vi "commander.vi"() -> ()   [LabVIEW 2012]
uses:
  <vilib>/Analysis/Matrix/Datatypes/RealMatrix.ctl
  G_VEH.vi
  G_SEN.vi
  G_PATH.vi
  G_DATA.vi
  G_LCM.vi
  <vilib>/Analysis/Matrix/Numeric/Conversions/Array To Matrix - RA2.vi
  <vilib>/Analysis/baseanly.llb/Real A x B.vi
  G_NAV.vi
  <vilib>/Analysis/Matrix/NI_Matrix.lvlib
  <vilib>/Analysis/NI_AALBase.lvlib
panel:
  in  "Boolean 2":bool
  out "Array":dbl[][](array[numeric])
  in  "Boolean":bool=TRUE
  out "LCM Recv Data":string
  out "GPS DATA 2":T1={"type"="None", "x_lcc"=-59.06772232055664, "y_lcc"=-26.082616806030273, "latdev"=0.0, "londev"=0.0, "sats"=0, "gps_l1_ranges"=0, "gps_l1_mask_ranges"=0, "gps_l2_mask_ranges"=0, "Heading"=89.78975677490234, "lon"=0.0, "lat"=0.0, "time"="None", "hgps"=89.78975677490234, "lag"=89.78975677490234, "MAP"="None"} {"lag" format="%#_5g"; "hgps" format="%#_5g"; "lat" format="%#_11g"; "lon" format="%#_11g"; "Heading" format="%#_5g"; "latdev" format="%#_4g"; "londev" format="%#_4g"}
  in  "LCM":bool
  in  "obs":bool
  in  "x":dbl
  in  "log":bool
  out "Waveform Chart 5":dbl(graph)
  in  "y":dbl min=-1.0 max=1.0 step=1.0
  out "x = 0?":bool
  out "timmer 2":u32
  out "timmer":u32
  out "Speed limit":dbl=8.0
  out "collision":bool
  out "Mission":i32=9
  in  "Load WPT":bool
  in  "Max. Vel.":dbl=20.0
  in  "RESET PATH":bool
  out "col":i16(graph)
  out "stop":bool
  in  "Reverse":bool
  in  "STOP":bool
  out "Waveform Chart 4":cluster{"auto":i16, "run":i16}(graph)={"auto"=1, "run"=0}
  out "Waveform Chart 3":T2(graph)={"Steer_input"=10.50986504720403, "Steer_output"=3.6, "handle"=10.50986504720403}
  out "Waveform Chart 2":T3(graph)={"VS_des"=4.606086314285715, "VS_can"=8.738, "VS_des"=5.0237113142857135}
  out "Heading":cluster{"Heading":dbl, "hgps":dbl}(graph)={"Heading"=269.76568785604456, "hgps"=270.2149981902155}
  out "XY Graph 2":cluster{"Y":dbl[], "Y":dbl[]}[](graph)=[{"Y"=[-241.57278442382812], "Y"=[-497.6172790527344]}, {"Y"=array[297 elements], "Y"=array[297 elements]}, {"Y"=array[297 elements], "Y"=array[297 elements]}, {"Y"=[-96.81030887093378], "Y"=[-438.1146154201037]}]
  out "Gauge":cluster{dbl, dbl, dbl}(knob)={4.606086314285715, 8.738, 5.0237113142857135} scale=-20.0..140.0
  out "Meter":cluster{dbl, dbl, dbl}(knob)={10.50986504720403, 3.6, 10.50986504720403} scale=-550.0..550.0
  out "XY Graph":cluster{"Y":dbl[], "Y":dbl[]}[](graph)=[{"Y"=[0.0], "Y"=[1000.0]}, {"Y"=[], "Y"=[]}, {"Y"=[], "Y"=[]}, {"Y"=[55.79381017995934], "Y"=[-143.41137512848826]}, {"Y"=[1.8243630881955273], "Y"=[-0.6091599202647308]}, {"Y"=[60.825233010671326, 56.37330625127248, 55.349089235151354, 59.801015994550255, 60.825233010671326], "Y"=[-144.72018116547483, -142.44414335187238, -144.44751039360185, -146.72354820720435, -144.72018116547483]}, {"Y"=[0.0, 2.210107140854234e-06, 8.840428449730098e-06, 1.9890964154001267e-05, 3.536171391260723e-05, 5.5252677611861145e-05, 7.956385525176302e-05, 0.00010829524660493917, 0.00014144685155770276, 0.0001790186695416196, 0.00022101070067037654, 0.00026742294460291305, 0.00031825540077079495, 0.00037350806894664856, 0.0004331809489031002, 0.0004972740399580289, 0.0005657873416566872, 0.0006387208537717015, 0.0007160745756209508, 0.0007978485066360008, 0.0008840426462484174, 0.0009746569938897665, 0.0010696915488779268, 0.0011691463105307776, 0.0012730212781661976, 0.001381316451102066, 0.0014940318285425747, 0.0016111674095782291, 0.0017327231935269083, 0.0018586991794791174, 0.001989095366525362, 0.00212391175364246, 0.002263148340148291, 0.0024068051247922995, 0.002554882106551304, 0.0027073792846294964, 0.002864296657776322, 0.003025634224741225, 0.003191391984614711, 0.0033615699362599116, 0.003536168078198898, 0.0037151864094084885, 0.003898624928524441, 0.004086483634296201, 0.004278762525359525, 0.004475461600350172, 0.0046765808579039, 0.004882120296656467, 0.0050920799150162566, 0.00530645971150534, 0.005525259684645789, 0.005748479832959674, 0.005976120154741693, 0.006208180648513917, 0.006444661312457356, 0.006685562145094082, 0.006930883144491418, 0.007180624309171435, 0.007434785636974084, 0.007693367126535122, 0.007956368775921874, 0.008223790583087975, 0.008495632546100751, 0.008771894663368585, 0.009052576932504053, 0.00933767935191554, 0.009627201919329309, 0.009921144632812684, 0.010219507490205615, 0.010522290489461739, 0.010829493628421005, 0.011141116904923365, 0.011457160316581394, 0.011777623861462416, 0.012102507536951634, 0.012431811341116372, 0.012765535271228146, 0.013103679325240591, 0.0134462435006526, 0.013793227794963059, 0.014144632205784546, 0.014500456730615952, 0.014860701366956164, 0.015225366112190386, 0.015594450963703821, 0.015967955919109045, 0.0163458809754502, 0.016728226130226176, 0.017114991380822175, 0.017506176724168654, 0.0179017821577645, 0.018301807678767545, 0.018706253284335617, 0.019115118971512857, 0.019528404737457095, 0.01994611057932616, 0.02036823649393682, 0.02079478247856059, 0.021225748530014243, 0.02166113464522823, 0.022100940821246695], "Y"=[0.0, 0.05249999993797367, 0.10499999950378934, 0.15749999832528905, 0.2099999960303148, 0.26249999224670867, 0.31499998660231265, 0.3674999787249688, 0.41999996824251923, 0.472499954782806, 0.5249999379736712, 0.577499917442957, 0.6299998928185055, 0.682499863728159, 0.7349998297997596, 0.7874997906611497, 0.8399997459401715, 0.8924996952646672, 0.9449996382624795, 0.9974995745614504, 1.0499995037894228, 1.1024994255742389, 1.1549993395437415, 1.2074992453257731, 1.2599991425481762, 1.3124990308387938, 1.3649989098254687, 1.4174987791360436, 1.4699986383983614, 1.5224984872402658, 1.574998325289599, 1.6274981521742047, 1.6799979675219257, 1.7324977709606055, 1.784997562118088, 1.837497340622216, 1.8899971061008334, 1.9424968581817836, 1.994996596492911, 2.047496320662059, 2.099996030317072, 2.152495725085793, 2.204995404596067, 2.2574950684757384, 2.309994716352652, 2.3624943478546507, 2.414993962609581, 2.467493560245286, 2.519993140389611, 2.5724927026704023, 2.6249922467155042, 2.6774917721527607, 2.7299912786100196, 2.7824907657151243, 2.834990233095921, 2.887489680380256, 2.939989107195975, 2.9924885131709242, 3.0449878979329497, 3.0974872611098974, 3.1499866023296144, 3.2024859212199472, 3.2549852174087435, 3.3074844905238483, 3.3599837401931105, 3.412482966044377, 3.464982167705495, 3.5174813448043127, 3.5699804969686775, 3.6224796238264374, 3.6749787250054404, 3.7274778001335362, 3.7799768488385714, 3.8324758707483966, 3.884974865490859, 3.9374738326938097, 3.989972771985096, 4.042471682992569, 4.094970565344078, 4.147469418667473, 4.199968242590603, 4.2524670367413195, 4.304965800747474, 4.3574645342369145, 4.409963236837495, 4.4624619081770645, 4.514960547883476, 4.567459155584579, 4.6199577309082285, 4.672456273482274, 4.724954782934569, 4.777453258892966, 4.829951700985317, 4.882450108839476, 4.934948482083297, 4.987446820344632, 5.039945123251335, 5.09244339043126, 5.144941621512262, 5.197439816122197, 5.249937973888915]}, {"Y"=[55.85492946607054, 56.300112183962334, 56.74529490185413, 57.19047761974598, 57.635660337637766, 58.08084305552956, 58.52602577342136, 58.97120849131315, 59.416391209205, 59.8615739270968, 60.306756644988596, 60.75193936288038, 61.197122080772175, 61.64230479866403, 62.087487516555825, 62.532670234447615, 62.97785295233941, 63.423035670231265, 63.86821838812306, 64.31340110601485, 64.75858382390665, 65.20376654179844, 65.64894925969023, 66.09413197758208, 66.53931469547388, 66.98449741336567, 67.42968013125746, 67.87486284914931, 68.3200455670411, 68.7652282849329, 69.2104110028247, 69.65559372071655, 70.10077643860835, 70.54595915650015, 70.99114187439193, 71.43632459228371, 71.88150731017556, 72.32669002806736, 72.77187274595916, 73.21705546385095], "Y"=[-143.26925304077835, -143.49687629901547, -143.72449955725253, -143.95212281548962, -144.17974607372668, -144.40736933196374, -144.63499259020085, -144.8626158484379, -145.090239106675, -145.3178623649121, -145.54548562314918, -145.7731088813862, -146.00073213962332, -146.22835539786038, -146.45597865609744, -146.68360191433456, -146.91122517257162, -147.1388484308087, -147.36647168904577, -147.59409494728285, -147.82171820551994, -148.04934146375703, -148.27696472199406, -148.50458798023115, -148.73221123846827, -148.9598344967053, -149.18745775494241, -149.4150810131795, -149.64270427141656, -149.87032752965362, -150.09795078789074, -150.3255740461278, -150.55319730436486, -150.78082056260195, -151.00844382083903, -151.23606707907612, -151.46369033731318, -151.6913135955503, -151.91893685378736, -152.14656011202442]}, {"Y"=[46.95734422441421, 47.0463827596022, 47.13542129479015, 47.224459829978144, 47.31349836516614, 47.40253690035408, 47.49157543554208, 47.58061397073008, 47.669652505918016, 47.75869104110601, 47.84772957629395, 47.936768111481946, 48.02580664666995, 48.11484518185789, 48.20388371704588, 48.292922252233886, 48.381960787421825, 48.47099932260982, 48.56003785779782, 48.64907639298576, 48.73811492817376, 48.827153463361746, 48.91619199854969, 49.00523053373769, 49.09426906892568, 49.18330760411363, 49.272346139301625, 49.361384674489564, 49.45042320967757, 49.53946174486556, 49.6285002800535, 49.717538815241504, 49.8065773504295, 49.89561588561743, 49.984654420805434, 50.07369295599343, 50.16273149118137, 50.251770026369364, 50.34080856155737, 50.429847096745306, 50.5188856319333, 50.607924167121304, 50.69696270230924, 50.78600123749724, 50.875039772685184, 50.96407830787318, 51.05311684306117, 51.142155378249115, 51.23119391343711, 51.320232448625106, 51.40927098381305, 51.49830951900105, 51.58734805418904, 51.67638658937698, 51.765425124564985, 51.85446365975298, 51.94350219494092, 52.03254073012892, 52.12157926531691, 52.21061780050485, 52.29965633569285, 52.38869487088079, 52.477733406068786, 52.56677194125679, 52.65581047644473, 52.74484901163272, 52.833887546820726, 52.922926082008665, 53.01196461719666, 53.10100315238466, 53.190041687572595, 53.27908022276059, 53.36811875794859, 53.45715729313653, 53.54619582832453, 53.635234363512524, 53.72427289870047, 53.813311433888465, 53.902349969076404, 53.99138850426441, 54.0804270394524, 54.16946557464034, 54.25850410982834, 54.34754264501633, 54.43658118020427, 54.525619715392274, 54.61465825058027, 54.70369678576821, 54.792735320956204, 54.88177385614421, 54.970812391332146, 55.05985092652014, 55.148889461708144, 55.23792799689608, 55.32696653208408, 55.41600506727202, 55.50504360246001, 55.59408213764801, 55.683120672835955, 55.77215920802395, 55.861197743211946, 55.95023627839994, 56.03927481358789, 56.12831334877588, 56.21735188396388, 56.306390419151825, 56.39542895433982, 56.48446748952781, 56.573506024715755, 56.66254455990375, 56.75158309509169, 56.84062163027969, 56.92966016546769, 57.01869870065563, 57.10773723584363, 57.196775771031625, 57.285814306219564, 57.37485284140757, 57.46389137659556, 57.552929911783494, 57.64196844697149, 57.73100698215949, 57.82004551734743, 57.90908405253543, 58.08716112291137, 58.176199658099364, 58.26523819328731, 58.354276728475305, 58.4433152636633, 58.53235379885125, 58.62139233403924, 58.71043086922723, 58.79946940441518, 58.88850793960317, 58.97754647479111, 59.06658500997911, 59.15562354516711, 59.24466208035505, 59.333700615543044, 59.42273915073105, 59.511777685918986, 59.60081622110698, 59.689854756294984, 59.778893291482916, 59.86793182667091, 59.956970361858914, 60.04600889704685, 60.13504743223485, 60.31312450261079, 60.402163037798786, 60.491201572986725, 60.58024010817473, 60.66927864336272, 60.75831717855066, 60.84735571373866, 60.93639424892665, 61.02543278411459, 61.114471319302595, 61.203509854490534, 61.29254838967853, 61.38158692486653, 61.47062546005447, 61.55966399524247, 61.64870253043047, 61.73774106561841, 61.826779600806404, 61.91581813599439, 62.00485667118234, 62.093895206370334, 62.18293374155833, 62.271972276746276, 62.36101081193427, 62.45004934712227, 62.53908788231021, 62.62812641749821, 62.71716495268615, 62.80620348787415, 62.895242023062146, 62.984280558250084, 63.07331909343808, 63.162357628626076, 63.251396163814015, 63.34043469900201, 63.42947323419001, 63.51851176937796, 63.60755030456595, 63.69658883975394, 63.78562737494189, 63.87466591012988, 63.96370444531783, 64.05274298050581, 64.14178151569382, 64.23082005088176, 64.31985858606976, 64.40889712125775, 64.4979356564457, 64.58697419163369, 64.76505126200964, 64.85408979719762, 64.94312833238557, 65.03216686757357, 65.12120540276156, 65.2102439379495, 65.29928247313751, 65.38832100832549, 65.47735954351344, 65.56639807870144, 65.65543661388938, 65.74447514907737, 65.83351368426537, 65.92255221945331, 66.0115907546413, 66.10062928982931, 66.18966782501724, 66.27870636020525, 66.36774489539324, 66.45678343058118, 66.54582196576918, 66.63486050095719, 66.72389903614511, 66.81293757133312, 66.9019761065211, 66.99101464170904, 67.08005317689705, 67.16909171208498, 67.25813024727299, 67.34716878246098, 67.43620731764892, 67.52524585283692, 67.61428438802493, 67.70332292321285, 67.79236145840086, 67.88139999358886, 67.97043852877678, 68.05947706396479, 68.14851559915279, 68.23755413434073, 68.32659266952872, 68.41563120471668, 68.50466973990466, 68.59370827509267, 68.6827468102806, 68.7717853454686, 68.8608238806566, 68.94986241584455, 69.03890095103253, 69.12793948622053, 69.21697802140848, 69.30601655659646, 69.39505509178447, 69.48409362697241, 69.5731321621604, 69.6621706973484, 69.75120923253635, 69.84024776772434, 69.92928630291229, 70.01832483810027, 70.10736337328828, 70.19640190847622, 70.2854404436642, 70.37447897885221, 70.46351751404015, 70.55255604922814, 70.64159458441614, 70.7306331196041, 70.81967165479207, 70.90871018998008, 70.99774872516802, 71.08678726035602, 71.17582579554401, 71.26486433073195, 71.35390286591995, 71.44294140110789, 71.5319799362959, 71.62101847148388, 71.71005700667183, 71.79909554185983, 71.88813407704782, 71.97717261223576, 72.06621114742377, 72.15524968261175, 72.2442882177997, 72.3333267529877, 72.42236528817568, 72.51140382336364, 72.60044235855163, 72.68948089373963, 72.77851942892757, 72.86755796411556, 72.9565964993035, 73.04563503449151, 73.13467356967949, 73.22371210486745, 73.31275064005544, 73.40178917524342, 73.49082771043138, 73.57986624561937], "Y"=[-138.89375124553214, -138.93927200180423, -138.98479275807625, -139.0303135143483, -139.07583427062036, -139.12135502689242, -139.16687578316444, -139.21239653943653, -139.25791729570855, -139.30343805198058, -139.34895880825266, -139.3944795645247, -139.44000032079677, -139.4855210770688, -139.53104183334085, -139.5765625896129, -139.62208334588496, -139.667604102157, -139.71312485842907, -139.7586456147011, -139.80416637097318, -139.8496871272452, -139.89520788351723, -139.9407286397893, -139.98624939606134, -140.0317701523334, -140.07729090860545, -140.1228116648775, -140.16833242114956, -140.2138531774216, -140.25937393369364, -140.30489468996572, -140.35041544623775, -140.39593620250977, -140.44145695878186, -140.48697771505388, -140.53249847132597, -140.578019227598, -140.62353998387005, -140.66906074014207, -140.71458149641416, -140.76010225268618, -140.80562300895826, -140.8511437652303, -140.89666452150234, -140.9421852777744, -140.98770603404643, -141.0332267903185, -141.07874754659053, -141.1242683028626, -141.16978905913462, -141.2153098154067, -141.26083057167872, -141.3063513279508, -141.35187208422283, -141.3973928404949, -141.44291359676694, -141.48843435303897, -141.53395510931105, -141.57947586558308, -141.62499662185516, -141.67051737812716, -141.71603813439924, -141.76155889067127, -141.80707964694335, -141.85260040321535, -141.89812115948743, -141.94364191575949, -141.9891626720315, -142.0346834283036, -142.08020418457562, -142.1257249408477, -142.1712456971197, -142.21676645339178, -142.2622872096638, -142.3078079659359, -142.3533287222079, -142.39884947847997, -142.44437023475203, -142.48989099102408, -142.53541174729614, -142.58093250356816, -142.62645325984025, -142.67197401611224, -142.71749477238433, -142.76301552865635, -142.80853628492844, -142.85405704120046, -142.89957779747255, -142.94509855374454, -142.99061931001663, -143.03614006628868, -143.0816608225607, -143.1271815788328, -143.17270233510482, -143.2182230913769, -143.2637438476489, -143.30926460392098, -143.354785360193, -143.4003061164651, -143.4458268727371, -143.4913476290092, -143.5368683852812, -143.58238914155328, -143.62790989782533, -143.67343065409736, -143.71895141036944, -143.76447216664147, -143.80999292291352, -143.85551367918555, -143.90103443545763, -143.94655519172966, -143.99207594800174, -144.03759670427374, -144.08311746054582, -144.12863821681785, -144.1741589730899, -144.21967972936199, -144.265200485634, -144.3107212419061, -144.3562419981781, -144.40176275445017, -144.4472835107222, -144.49280426699428, -144.58384577953836, -144.6293665358104, -144.67488729208247, -144.72040804835453, -144.76592880462653, -144.81144956089864, -144.85697031717064, -144.90249107344272, -144.94801182971474, -144.99353258598683, -145.03905334225882, -145.0845740985309, -145.13009485480293, -145.17561561107502, -145.22113636734704, -145.2666571236191, -145.31217787989118, -145.35769863616318, -145.40321939243526, -145.4487401487073, -145.49426090497937, -145.5397816612514, -145.58530241752348, -145.63082317379548, -145.7218646863396, -145.76738544261164, -145.8129061988837, -145.85842695515572, -145.90394771142783, -145.94946846769983, -145.9949892239719, -146.04050998024394, -146.08603073651602, -146.13155149278802, -146.1770722490601, -146.22259300533213, -146.2681137616042, -146.31363451787624, -146.3591552741483, -146.40467603042035, -146.45019678669237, -146.49571754296446, -146.54123829923648, -146.58675905550857, -146.6322798117806, -146.67780056805265, -146.72332132432467, -146.76884208059676, -146.81436283686878, -146.85988359314084, -146.9054043494129, -146.95092510568492, -146.99644586195703, -147.04196661822903, -147.0874873745011, -147.13300813077313, -147.17852888704522, -147.22404964331722, -147.2695703995893, -147.31509115586132, -147.3606119121334, -147.40613266840543, -147.4516534246775, -147.49717418094954, -147.54269493722157, -147.58821569349365, -147.63373644976568, -147.67925720603776, -147.72477796230976, -147.77029871858184, -147.81581947485387, -147.86134023112595, -147.90686098739798, -147.9979024999421, -148.0434232562141, -148.08894401248617, -148.13446476875822, -148.17998552503028, -148.22550628130233, -148.27102703757438, -148.3165477938464, -148.3620685501185, -148.40758930639052, -148.45311006266255, -148.49863081893463, -148.54415157520666, -148.58967233147874, -148.63519308775076, -148.6807138440228, -148.72623460029487, -148.77175535656693, -148.81727611283895, -148.86279686911104, -148.90831762538306, -148.95383838165512, -148.99935913792717, -149.0448798941992, -149.09040065047128, -149.1359214067433, -149.18144216301536, -149.22696291928742, -149.27248367555944, -149.31800443183153, -149.36352518810358, -149.4090459443756, -149.4545667006477, -149.50008745691972, -149.54560821319174, -149.59112896946382, -149.63664972573585, -149.68217048200793, -149.72769123827996, -149.77321199455199, -149.81873275082407, -149.86425350709612, -149.90977426336815, -149.95529501964023, -150.00081577591226, -150.0463365321843, -150.09185728845637, -150.1373780447284, -150.18289880100048, -150.2284195572725, -150.27394031354456, -150.3194610698166, -150.36498182608864, -150.4105025823607, -150.45602333863278, -150.5015440949048, -150.54706485117688, -150.5925856074489, -150.63810636372094, -150.68362711999302, -150.72914787626505, -150.7746686325371, -150.82018938880915, -150.86571014508118, -150.91123090135326, -150.9567516576253, -151.00227241389734, -151.04779317016943, -151.09331392644145, -151.13883468271348, -151.18435543898556, -151.2298761952576, -151.27539695152967, -151.3209177078017, -151.36643846407375, -151.4119592203458, -151.45747997661783, -151.5030007328899, -151.54852148916194, -151.594042245434, -151.63956300170608, -151.6850837579781, -151.73060451425013, -151.77612527052221, -151.82164602679424, -151.8671667830663, -151.91268753933835, -151.95820829561038, -152.00372905188246, -152.04924980815449, -152.09477056442654, -152.14029132069862, -152.18581207697065, -152.23133283324267, -152.27685358951476, -152.32237434578678, -152.36789510205887, -152.4134158583309, -152.45893661460295, -152.504457370875]}, {"Y"=[], "Y"=[]}, {"Y"=[], "Y"=[]}, {"Y"=[], "Y"=[]}, {"Y"=[-16.5, -15.25, -15.0, -13.5, -13.25, -13.25, -13.25, -13.0, -13.0, -12.75, -12.75, -12.75, -12.75, -12.75, -12.75, -12.75, -12.5, -12.5, -12.5, -12.5, -12.5, -12.5, -12.25, -12.25, -12.25, -12.25, -12.25, -12.25, -12.0, -12.0, -12.0, -11.75, -11.75, -11.75, -11.5, -11.5, -11.5, -11.5, -11.5, -11.25, -10.75, -10.75, -10.5, -10.5, -10.25, -10.25, -10.0, -10.0, -10.0, -10.0, -10.0, -9.75, -9.75, -9.75, -9.75, -9.75, -9.75, -9.75, -9.75, -9.75, -9.75, -9.5, -9.5, -9.5, -9.5, -9.5, -9.5, -9.5, -9.5, -9.5, -9.5, -9.5, -9.5, -9.5, -9.5, -9.5, -9.5, -9.5, -9.5, -9.5, -9.25, -9.25, -9.25, -9.25, -9.25, -9.25, -9.25, -9.25, -9.25, -9.25, -9.25, -9.25, -9.25, -9.25, -9.25, -9.25, -9.25, -9.25, -9.25, -9.25, -9.25, -9.25, -9.0, -9.0, -9.0, -9.0, -9.0, -9.0, -9.0, -9.0, -9.0, -9.0, -9.0, -9.0, -9.0, -9.0, -9.0, -9.0, -9.0, -9.0, -9.0, -9.0, -9.0, -9.0, -9.0, -9.0, -9.0, -9.0, -8.75, -8.75, -8.75, -8.75, -8.75, -8.75, -8.75, -8.75, -8.75, -8.75, -8.75, -8.75, -8.75, -8.75, -8.75, -8.75, -8.75, -8.75, -8.75, -8.75, -8.75, -8.75, -8.75, -8.75, -8.75, -8.75, -8.75, -8.75, -8.75, -8.75, -8.75, -8.75, -8.75, -8.75, -8.75, -8.75, -8.75, -8.5, -8.5, -8.5, -8.5, -8.5, -8.5, -8.5, -8.5, -8.5, -8.5, -8.5, -8.5, -8.5, -8.5, -8.5, -8.5, -8.5, -8.5, -8.5, -8.5, -8.5, -8.5, -8.5, -8.5, -8.5, -8.5, -8.5, -8.5, -8.5, -8.5, -8.5, -8.5, -8.5, -8.5, -8.5, -8.5, -8.25, -8.25, -8.25, -8.25, -8.25, -8.25, -8.25, -8.25, -8.25, -8.25, -8.25, -8.25, -8.25, -8.25, -8.25, -8.25, -8.25, -8.25, -8.25, -8.25, -8.25, -8.25, -8.25, -8.25, -8.25, -8.25, -8.25, -8.25, -8.25, -8.25, -8.25, -8.25, -8.25, -8.0, -8.0, -8.0, -8.0, -8.0, -8.0, -8.0, -8.0, -8.0, -8.0, -8.0, -8.0, -8.0, -8.0, -8.0, -8.0, -8.0, -8.0, -8.0, -8.0, -8.0, -8.0, -8.0, -8.0, -8.0, -7.75, -7.75, -7.75, -7.75, -7.75, -7.75, -7.75, -7.75, -7.75, -7.75, -7.75, -7.75, -7.75, -7.75, -7.75, -7.75, -7.75, -7.75, -7.75, -7.75, -7.75, -7.75, -7.75, -7.75, -7.75, -7.75, -7.5, -7.5, -7.5, -7.5, -7.5, -7.5, -7.5, -7.5, -7.5, -7.5, -7.5, -7.5, -7.5, -7.5, -7.5, -7.5, -7.5, -7.5, -7.5, -7.5, -7.5, -7.5, -7.5, -7.5, -7.5, -7.25, -7.25, -7.25, -7.25, -7.25, -7.25, -7.25, -7.25, -7.25, -7.25, -7.25, -7.25, -7.25, -7.25, -7.25, -7.25, -7.25, -7.25, -7.25, -7.25, -7.25, -7.25, -7.25, -7.0, -7.0, -7.0, -7.0, -7.0, -7.0, -7.0, -7.0, -7.0, -7.0, -7.0, -7.0, -7.0, -7.0, -7.0, -7.0, -7.0, -7.0, -7.0, -6.75, -6.75, -6.75, -6.75, -6.75, -6.75, -6.75, -6.75, -6.75, -6.75, -6.75, -6.75, -6.75, -6.75, -6.75, -6.75, -6.75, -6.75, -6.75, -6.75, -6.75, -6.75, -6.75, -6.5, -6.5, -6.5, -6.5, -6.5, -6.5, -6.5, -6.5, -6.5, -6.5, -6.5, -6.5, -6.5, -6.5, -6.5, -6.5, -6.5, -6.5, -6.5, -6.5, -6.5, -6.5, -6.5, -6.5, -6.5, -6.5, -6.5, -6.5, -6.5, -6.5, -6.25, -6.25, -6.25, -6.25, -6.25, -6.25, -6.25, -6.25, -6.25, -6.25, -6.25, -6.25, -6.25, -6.25, -6.25, -6.25, -6.25, -6.0, -6.0, -6.0, -6.0, -6.0, -6.0, -6.0, -6.0, -6.0, -6.0, -6.0, -5.75, -5.75, -5.75, -5.75, -5.75, -5.75, -5.75, -5.75, -5.75, -5.75, -5.5, -5.25, -5.0, -4.75, -4.5, -4.5, -4.25, -4.25, -4.0, -4.0, -3.75, -3.75, -3.5, -3.5, -3.25, -3.25, -3.25, -3.25, -3.0, -3.0, 2.0, 2.0, 2.0, 2.0, 2.0, 2.0, 2.0, 2.25, 2.25, 2.25, 2.25, 2.25, 2.25, 2.25, 2.25, 2.25, 2.25, 2.25, 2.25, 2.25, 2.25, 2.25, 2.25, 2.25, 2.25, 2.25, 2.25, 2.25, 2.25, 2.5, 2.5, 2.5, 2.5, 2.5, 2.5, 2.5, 2.5, 2.5, 2.5, 2.5, 2.5, 2.5, 2.5, 2.5, 2.5, 2.5, 2.5, 2.5, 2.5, 2.5, 2.5, 2.5, 2.5, 2.5, 2.5, 2.5, 2.5, 2.5, 2.5, 2.5, 2.5, 2.5, 2.5, 2.5, 2.5, 2.5, 2.5, 2.5, 2.5, 2.5, 2.5, 2.75, 2.75, 2.75, 2.75, 2.75, 2.75, 2.75, 2.75, 2.75, 2.75, 2.75, 2.75, 2.75, 2.75, 2.75, 2.75, 2.75, 2.75, 2.75, 2.75, 2.75, 2.75, 2.75, 2.75, 2.75, 2.75, 2.75, 2.75, 2.75, 2.75, 2.75, 2.75, 2.75, 2.75, 2.75, 2.75, 2.75, 2.75, 2.75, 2.75, 2.75, 2.75, 2.75, 2.75, 2.75, 2.75, 2.75, 2.75, 2.75, 2.75, 3.0, 3.0, 3.0, 3.0, 3.0, 3.0, 3.0, 3.0, 3.0, 3.0, 3.0, 3.0, 3.0, 3.0, 3.0, 3.0, 3.0, 3.0, 3.0, 3.0, 3.0, 3.0, 3.0, 3.0, 3.0, 3.0, 3.0, 3.0, 3.0, 3.0, 3.0, 3.0, 3.0, 3.0, 3.0, 3.0, 3.0, 3.0, 3.0, 3.0, 3.0, 3.0, 3.0, 3.0, 3.0, 3.0, 3.0, 3.25, 3.25, 3.25, 3.25, 3.25, 3.25, 3.25, 3.25, 3.25, 3.25, 3.25, 3.25, 3.25, 3.25, 3.25, 3.25, 3.25, 3.25, 3.25, 3.25, 3.25, 3.25, 3.25, 3.25, 3.25, 3.25, 3.25, 3.25, 3.25, 3.25, 3.25, 3.25, 3.25, 3.25, 3.25, 3.25, 3.25, 3.25, 3.25, 3.25, 3.25, 3.25, 3.25, 3.25, 3.25, 3.25, 3.25, 3.25, 3.25, 3.25, 3.25, 3.25, 3.25, 3.5, 3.5, 3.5, 3.5, 3.5, 3.5, 3.5, 3.5, 3.5, 3.5, 3.5, 3.5, 3.5, 3.5, 3.5, 3.5, 3.5, 3.5, 3.5, 3.5, 3.5, 3.5, 3.5, 3.5, 3.5, 3.5, 3.5, 3.5, 3.5, 3.5, 3.5, 3.5, 3.5, 3.5, 3.5, 3.5, 3.5, 3.5, 3.5, 3.5, 3.5, 3.5, 3.5, 3.5, 3.5, 3.5, 3.5, 3.5, 3.5, 3.5, 3.5, 3.5, 3.5, 3.5, 3.5, 3.5, 3.5, 3.75, 3.75, 3.75, 3.75, 3.75, 3.75, 3.75, 3.75, 3.75, 3.75, 3.75, 3.75, 3.75, 3.75, 3.75, 3.75, 3.75, 3.75, 3.75, 3.75, 3.75, 3.75, 3.75, 3.75, 3.75, 3.75, 3.75, 3.75, 3.75, 3.75, 3.75, 3.75, 3.75, 3.75, 3.75, 3.75, 3.75, 4.0, 4.0, 4.0, 4.0, 4.0, 4.0, 4.0, 4.0, 4.0, 4.0, 4.0, 4.0, 4.0, 4.0, 4.0, 4.0, 4.0, 4.0, 4.0, 4.0, 4.0, 4.0, 4.0, 4.0, 4.0, 4.0, 4.0, 4.0, 4.0, 4.0, 4.0, 4.0, 4.0, 4.0, 4.0, 4.0, 4.25, 4.25, 4.25, 4.25, 4.25, 4.25, 4.25, 4.25, 4.25, 4.25, 4.25, 4.25, 4.25, 4.25, 4.25, 4.25, 4.25, 4.25, 4.25, 4.25, 4.25, 4.25, 4.25, 4.25, 4.25, 4.25, 4.25, 4.25, 4.25, 4.25, 4.25, 4.25, 4.25, 4.25, 4.25, 4.25, 4.25, 4.25, 4.25, 4.25, 4.25, 4.25, 4.25, 4.5, 4.5, 4.5, 4.5, 4.5, 4.5, 4.5, 4.5, 4.5, 4.5, 4.5, 4.5, 4.5, 4.5, 4.5, 4.5, 4.5, 4.5, 4.5, 4.5, 4.5, 4.5, 4.5, 4.5, 4.5, 4.5, 4.5, 4.75, 4.75, 4.75, 4.75, 4.75, 4.75, 4.75, 4.75, 4.75, 4.75, 4.75, 4.75, 4.75, 4.75, 4.75, 4.75, 4.75, 4.75, 4.75, 4.75, 4.75, 4.75, 4.75, 4.75, 4.75, 4.75, 4.75, 4.75, 4.75, 5.0, 5.0, 5.0, 5.0, 5.0, 5.0, 5.0, 5.0, 5.0, 5.0, 5.0, 5.0, 5.0, 5.0, 5.0, 5.0, 5.0, 5.0, 5.0, 5.0, 5.0, 5.25, 5.25, 5.25, 5.25, 5.25, 5.25, 5.25, 5.25, 5.25, 5.25, 5.25, 5.25, 5.25, 5.25, 5.5, 5.5, 5.5, 5.5, 5.5, 5.5, 5.5, 5.5, 5.5, 5.5, 5.5, 5.5, 5.75, 5.75, 5.75, 5.75, 5.75, 5.75, 5.75, 5.75, 5.75, 5.75, 5.75, 5.75, 5.75, 5.75, 5.75, 5.75, 5.75, 6.0, 6.0, 6.0, 6.0, 6.0, 6.0, 6.0, 6.0, 6.0, 6.0, 6.0, 6.25, 6.25, 6.25, 6.25, 6.25, 6.25, 6.25, 6.25, 6.5, 6.5, 6.5, 6.5, 6.5, 6.5, 6.5, 6.5, 6.5, 6.75, 6.75, 6.75, 6.75, 7.0, 7.0, 7.0, 7.25, 7.25, 7.25, 7.25, 7.25, 7.25, 7.25, 7.5, 7.5, 8.0, 8.0, 8.0, 8.0, 8.0, 8.25, 8.25, 8.5, 8.5, 8.5, 8.75, 8.75, 8.75, 8.75, 8.75, 9.0, 9.0, 9.0, 9.0, 9.0, 9.0, 9.25, 9.25, 9.25, 9.25, 9.25, 9.25, 9.5, 9.5, 9.5, 9.5, 9.5, 9.5, 9.75, 9.75, 9.75, 10.0, 10.0, 10.0, 10.0, 10.25, 10.25, 10.5, 10.5, 10.5, 10.75, 10.75, 10.75, 10.75, 11.0, 11.0, 11.0, 11.0, 11.0, 11.25, 11.25, 11.25, 11.25, 11.25, 11.25, 11.25, 11.25, 11.25, 11.25, 11.5, 11.5, 11.5, 11.5, 11.5, 11.5, 11.5, 11.5, 11.5, 11.5, 11.5, 11.5, 11.5, 11.5, 11.5, 11.75, 11.75, 11.75, 11.75, 11.75, 11.75, 11.75, 11.75, 11.75, 11.75, 11.75, 11.75, 11.75, 11.75, 11.75, 11.75, 11.75, 11.75, 11.75, 11.75, 12.0, 12.0, 12.0, 12.0, 12.0, 12.0, 12.0, 12.0, 12.0, 12.0, 12.0, 12.0, 12.0, 12.0, 12.0, 12.0, 12.0, 12.0, 12.0, 12.0, 12.0, 12.0, 12.0, 12.0, 12.0, 12.0, 12.0, 12.25, 12.25, 12.25, 12.25, 12.25, 12.25, 12.25, 12.25, 12.25, 12.25, 12.25, 12.25, 12.25, 12.25, 12.25, 12.25, 12.5, 12.5, 12.5, 12.5, 12.5, 12.5, 12.5, 12.5, 12.5, 12.5, 12.5, 12.5, 12.5, 12.75, 12.75, 12.75, 12.75, 12.75, 12.75, 12.75, 12.75, 12.75, 12.75, 13.0, 13.0, 13.0, 13.0, 13.0, 13.0, 13.0, 13.0, 13.0, 13.0, 13.0, 13.0, 13.0, 13.0, 13.0, 13.0, 13.0, 13.0, 13.0, 13.0, 13.0, 13.0, 13.0, 13.25, 13.25, 13.25, 13.25, 13.25, 13.25, 13.25, 13.25, 13.25, 13.25, 13.25, 13.25, 13.25, 13.25, 13.25, 13.25, 13.25, 13.25, 13.25, 13.5, 13.5, 13.5, 13.5, 13.5, 13.5, 13.5, 13.5, 13.5, 13.5, 13.75, 13.75, 13.75, 13.75, 13.75, 13.75, 13.75, 13.75, 13.75, 14.0, 14.0, 14.0, 14.0, 14.5, 14.75, 15.5, 15.75, 16.0, 19.25, 19.25, 19.25, 19.5, 19.5, 19.75, 22.25, 22.25, 22.25, 22.5, 22.5, 22.5, 22.75, 22.75, 22.75, 22.75, 23.0, 23.0, 23.0, 23.25, 23.25, 23.25, 23.5, 23.5, 23.5, 23.5, 23.5, 23.5, 23.75, 23.75, 23.75, 23.75, 23.75, 23.75, 23.75, 23.75, 23.75, 23.75, 23.75, 24.0, 24.0, 24.0, 24.0, 24.0, 24.0, 24.0, 24.25, 24.25, 24.5], "Y"=[46.5, 46.5, 46.5, 2.75, 0.5, 2.75, 17.0, 0.75, 17.25, -6.5, -2.25, -1.75, 0.5, 0.75, 1.0, 3.75, -6.5, 0.75, 4.0, 4.25, 17.25, 21.5, -6.75, -6.5, -1.75, 17.25, 21.5, 22.25, -6.75, 21.75, 22.0, -6.5, 11.25, 22.0, 10.5, 10.75, 11.0, 11.5, 11.75, -6.0, 3.75, 8.25, -1.0, 8.25, -1.25, -1.0, -7.0, -1.25, 2.75, 3.0, 3.5, -10.75, -10.5, -10.0, -9.5, -9.25, -8.25, -6.75, -1.25, 3.0, 3.25, -20.5, -15.5, -15.25, -14.75, -10.5, -10.25, -10.0, -9.75, -9.25, -9.0, -8.75, -8.25, -8.0, -7.75, -7.5, -1.0, 0.5, 1.5, 2.75, -20.25, -18.25, -17.75, -17.5, -17.0, -15.75, -15.5, -10.75, -10.25, -9.5, -9.0, -8.75, -8.25, -8.0, -7.75, 0.75, 1.0, 1.25, 2.25, 3.5, 7.25, 7.5, -19.0, -17.5, -17.25, -10.5, -10.25, -10.0, -9.25, -9.0, -8.75, -8.25, -8.0, -7.25, -7.0, -6.75, -4.75, -4.5, -4.25, 0.75, 1.0, 1.25, 1.75, 2.25, 2.5, 2.75, 3.5, 7.5, -17.5, -12.75, -12.0, -11.75, -10.5, -9.75, -9.5, -9.25, -9.0, -8.75, -8.5, -8.25, -8.0, -7.75, -7.5, -7.0, -6.75, -4.75, -4.5, -3.75, -3.25, -3.0, -1.5, -0.5, -0.25, 0.0, 0.25, 1.75, 2.5, 2.75, 4.25, 4.75, 5.5, 5.75, 6.25, 7.5, 7.75, -13.25, -13.0, -12.75, -12.0, -11.75, -8.25, -8.0, -7.0, -6.75, -5.5, -5.0, -4.75, -4.5, -4.0, -3.75, -3.25, -3.0, -2.75, -2.0, -1.75, -1.5, -1.0, -0.5, -0.25, 0.0, 0.25, 0.5, 0.75, 1.75, 2.0, 4.0, 4.25, 4.75, 5.75, 6.0, 6.25, -17.5, -12.75, -12.0, -11.5, -10.25, -8.25, -8.0, -7.75, -5.5, -4.75, -4.0, -3.75, -3.5, -3.25, -3.0, -2.75, -2.5, -2.25, -2.0, -1.75, -1.5, -0.75, -0.5, -0.25, 0.0, 0.25, 0.5, 2.25, 4.5, 4.75, 5.75, 6.0, 6.25, -13.5, -13.25, -13.0, -7.75, -5.75, -5.5, -5.25, -5.0, -4.75, -4.5, -3.75, -3.5, -3.25, -2.25, -2.0, -1.75, -1.5, -1.25, -0.75, -0.5, -0.25, 0.0, 0.25, 0.5, 0.75, -13.25, -12.5, -6.0, -5.75, -5.25, -5.0, -4.75, -4.5, -4.25, -3.25, -2.5, -2.25, -2.0, -1.75, -1.5, -1.25, -0.75, -0.5, -0.25, 0.0, 0.25, 0.5, 4.0, 4.25, 7.75, 8.0, -14.0, -13.25, -13.0, -8.0, -5.25, -5.0, -4.75, -3.75, -3.0, -2.0, -1.75, -1.5, -1.25, -0.5, -0.25, 0.25, 0.5, 0.75, 1.0, 1.25, 1.5, 2.25, 2.5, 3.75, 9.25, -7.75, -7.25, -7.0, -6.75, -6.5, -6.25, -6.0, -5.75, -5.5, -5.25, -5.0, -3.5, -1.75, -1.5, -1.25, -0.5, -0.25, 1.0, 1.25, 1.75, 2.5, 5.75, 8.5, -9.0, -8.0, -7.75, -7.0, -6.75, -6.5, -5.5, -5.25, -5.0, -2.0, -1.75, 1.25, 1.5, 2.5, 4.0, 4.25, 4.5, 6.0, 8.5, -9.25, -9.0, -7.5, -7.25, -5.75, -5.5, -2.75, -2.5, -1.0, -0.75, -0.5, -0.25, 0.0, 1.0, 1.25, 1.75, 2.75, 3.0, 4.5, 4.75, 5.75, 6.0, 6.25, -20.0, -8.0, -7.5, -7.25, -4.5, -4.25, -3.25, -3.0, -2.75, -2.5, -1.25, -1.0, -0.75, -0.5, 2.25, 2.5, 2.75, 3.0, 3.25, 3.5, 3.75, 4.0, 4.25, 4.5, 4.75, 5.0, 5.25, 5.5, 5.75, 6.0, -20.25, -20.0, -14.0, -13.75, -8.0, -7.75, -7.25, -5.0, -4.75, -4.5, -3.5, -3.25, -3.0, -2.0, -1.75, -1.5, 3.0, -20.0, -14.0, -13.75, -8.0, -7.75, -7.5, -7.25, -5.0, -2.0, -1.75, -1.5, -20.5, -20.25, -14.25, -8.0, -7.75, -7.5, -2.0, -1.75, -1.5, 3.0, 3.0, 3.0, 3.0, 3.0, 3.0, 20.75, 3.0, 20.75, 3.0, 20.75, 3.0, 20.75, 3.0, 20.75, 3.0, 21.0, 22.0, 22.25, 3.0, 22.25, -8.25, -8.0, -7.25, -2.75, -2.5, -2.25, -2.0, -20.5, -14.5, -14.25, -8.5, -8.25, -8.0, -7.75, -7.25, -4.5, -4.0, -3.5, -3.25, -3.0, -2.5, -2.25, -2.0, -1.5, -1.25, -1.0, 4.75, 6.0, 6.25, -20.5, -20.25, -14.25, -8.25, -8.0, -7.75, -5.0, -4.5, -4.25, -4.0, -3.75, -3.5, -3.25, -3.0, -2.75, -2.5, -2.25, -2.0, -1.75, -1.5, -1.25, -1.0, -0.75, 0.75, 1.75, 2.0, 2.25, 2.5, 2.75, 3.0, 3.25, 3.5, 3.75, 4.0, 5.0, 5.25, 5.5, 5.75, 6.25, 6.5, 6.75, 7.0, -20.5, -20.25, -14.25, -8.25, -7.75, -4.75, -4.5, -4.25, -4.0, -3.75, -3.5, -3.25, -3.0, -2.75, -2.5, -2.0, -1.75, -1.5, -1.25, -1.0, -0.75, -0.5, 0.25, 0.5, 0.75, 1.0, 1.25, 1.5, 1.75, 2.0, 2.25, 2.5, 2.75, 3.25, 3.5, 3.75, 4.0, 4.25, 4.5, 4.75, 5.0, 5.25, 5.5, 5.75, 6.0, 6.25, 6.5, 6.75, 7.0, 7.25, -20.25, -7.75, -5.25, -4.5, -4.25, -4.0, -3.75, -3.5, -3.25, -2.75, -2.5, -2.25, -2.0, -1.75, -1.5, -1.25, -1.0, -0.75, -0.5, -0.25, 0.0, 0.25, 0.5, 0.75, 1.0, 1.25, 1.5, 1.75, 2.0, 2.25, 2.5, 2.75, 4.25, 4.5, 4.75, 5.0, 5.25, 5.5, 5.75, 6.0, 6.25, 6.5, 6.75, 7.0, 7.5, 9.5, 10.75, -20.5, -7.5, -6.75, -6.0, -5.75, -5.0, -4.75, -4.5, -4.25, -4.0, -3.25, -3.0, -2.75, -2.5, -2.0, -1.75, -1.5, -1.25, -1.0, -0.75, -0.5, -0.25, 0.0, 0.25, 0.5, 0.75, 1.0, 1.25, 1.5, 1.75, 2.0, 2.25, 2.5, 2.75, 3.0, 4.5, 4.75, 5.0, 5.25, 5.5, 5.75, 6.0, 6.25, 6.5, 6.75, 7.0, 7.25, 9.25, 9.5, 10.75, 11.0, 12.25, 12.75, -7.75, -7.5, -6.75, -6.5, -5.75, -5.5, -5.25, -4.75, -4.25, -4.0, -3.5, -3.0, -2.75, -2.25, -2.0, -1.75, -1.5, -1.25, -1.0, -0.75, -0.5, -0.25, 0.0, 0.25, 0.5, 0.75, 1.0, 1.25, 1.5, 1.75, 2.0, 2.25, 2.5, 2.75, 3.0, 4.75, 5.0, 5.25, 5.5, 5.75, 6.0, 6.5, 6.75, 7.0, 8.75, 9.0, 9.25, 10.25, 10.75, 11.0, 11.25, 12.25, 12.5, 12.75, 13.0, 13.25, 13.75, -8.75, -7.5, -6.5, -6.25, -5.5, -5.0, -4.75, -4.5, -4.25, -4.0, -2.25, -1.75, -1.5, -1.25, -1.0, -0.75, -0.5, -0.25, 0.0, 0.25, 0.5, 1.0, 1.25, 1.5, 1.75, 2.0, 2.25, 2.5, 2.75, 3.0, 3.25, 9.75, 11.0, 11.25, 12.25, 12.5, 13.0, -8.5, -7.5, -6.75, -6.5, -5.5, -5.25, -4.25, -4.0, -3.25, -3.0, -2.75, -2.5, -2.25, -1.75, -1.5, -1.25, -1.0, -0.75, -0.5, -0.25, 0.0, 0.25, 0.5, 0.75, 1.0, 1.25, 1.5, 1.75, 2.0, 2.25, 2.5, 2.75, 3.0, 12.5, 13.0, 13.25, -9.75, -9.5, -9.25, -8.75, -8.5, -8.25, -7.75, -7.5, -7.25, -7.0, -6.75, -6.5, -6.25, -6.0, -5.75, -5.0, -4.25, -3.0, -2.75, -2.5, -2.25, -1.75, -1.5, 0.0, 0.25, 0.5, 0.75, 1.0, 1.25, 1.5, 1.75, 2.0, 2.5, 2.75, 3.0, 3.25, 11.0, 11.25, 11.5, 12.0, 12.25, 12.5, 13.0, -10.0, -9.0, -8.75, -8.5, -8.25, -7.5, -7.25, -6.5, -6.0, -5.75, -4.5, -4.25, -4.0, -3.0, 0.25, 0.5, 0.75, 1.0, 2.5, 2.75, 3.0, 3.5, 11.5, 11.75, 12.0, 12.25, 12.75, -11.25, -10.75, -10.0, -9.5, -9.25, -9.0, -8.75, -8.0, -7.25, -7.0, -6.5, -6.25, -6.0, -5.75, -5.5, -4.75, -4.5, -4.25, -4.0, -3.75, 2.25, 2.5, 2.75, 3.0, 3.5, 6.75, 11.25, 11.5, 12.0, -12.25, -9.0, -8.75, -6.5, -6.25, -6.0, -5.75, -5.5, -5.25, -5.0, -4.75, -4.25, -4.0, -3.75, -3.5, 1.25, 2.5, 2.75, 3.25, 6.75, 12.0, -9.0, -8.75, -8.5, -7.0, -5.75, -5.5, -4.25, -3.5, -3.25, -3.0, -0.75, 2.0, 2.25, 12.0, -10.75, -9.0, -8.25, -3.25, -3.0, 2.0, 2.25, 2.5, 4.25, 5.75, 12.0, 13.0, -9.0, -3.5, 1.0, 1.25, 1.5, 1.75, 2.25, 2.5, 2.75, 3.25, 5.5, 5.75, 8.25, 8.5, 8.75, 9.0, 9.25, -9.0, -8.75, 1.5, 1.75, 3.25, 3.5, 5.5, 5.75, 6.25, 8.25, 9.0, -9.0, -8.75, 1.75, 3.25, 3.75, 5.75, 9.0, 9.5, -17.25, 1.5, 1.75, 3.25, 4.75, 5.5, 6.0, 6.25, 6.75, 4.5, 4.75, 5.5, 6.25, 4.5, 4.75, 5.75, 4.5, 6.25, 8.75, 9.0, 10.25, 10.5, 17.0, 4.0, 17.0, 1.5, 6.75, 10.75, 11.0, 17.5, 0.0, 17.5, 3.25, 17.25, 17.5, 0.25, 3.0, 3.25, 11.25, 11.5, -0.5, 6.75, 11.25, 11.5, 12.25, 35.5, -11.25, 12.0, 12.25, 12.75, 17.0, 35.5, -13.0, -12.25, -10.75, 12.0, 12.25, 17.0, 16.5, 16.75, 28.5, 16.25, 16.5, 28.25, 28.75, 28.0, 28.5, 2.25, 28.0, 28.25, 2.0, 2.5, 3.25, 8.0, 2.75, 3.25, 8.0, 8.25, 15.75, -7.75, -7.5, -5.25, -4.75, -2.25, 5.25, 8.0, 8.25, 15.25, 15.5, -9.25, -7.25, -4.75, -3.5, -3.0, -2.5, 2.5, 4.0, 4.25, 4.5, 4.75, 7.0, 7.75, 8.75, 9.0, -7.75, 1.0, 1.5, 2.25, 2.5, 2.75, 3.0, 3.25, 3.5, 3.75, 4.0, 4.25, 4.5, 4.75, 5.0, 5.25, 6.25, 8.0, 10.5, 28.75, -11.25, -7.25, 1.5, 1.75, 2.0, 2.25, 2.5, 2.75, 3.0, 3.25, 3.5, 3.75, 4.0, 4.25, 4.75, 5.0, 5.25, 5.5, 5.75, 6.0, 6.25, 6.5, 7.0, 7.25, 7.5, 7.75, 14.25, 1.75, 2.0, 2.5, 3.25, 3.75, 4.0, 5.75, 6.0, 6.25, 6.5, 6.75, 7.5, 9.25, 13.0, 13.25, 14.0, 1.75, 2.0, 2.5, 3.0, 3.25, 3.5, 6.0, 8.0, 8.25, 9.25, 10.25, 13.5, 13.75, -1.75, -1.5, -1.25, 3.25, 3.5, 4.0, 7.0, 8.0, 9.0, 13.0, -9.5, -5.0, -4.5, -4.25, -4.0, -3.75, -2.0, -1.75, -1.5, -1.25, -1.0, -0.75, -0.5, -0.25, 0.0, 0.25, 6.0, 7.5, 8.75, 9.5, 10.25, 12.25, 12.5, -5.5, -5.25, -5.0, -4.75, -4.5, -4.0, -3.75, -3.5, -2.0, -1.75, -1.0, -0.25, 0.25, 1.0, 1.25, 1.5, 7.5, 10.5, 10.75, -6.75, -6.5, -6.25, -6.0, -5.75, -5.5, 1.0, 1.25, 5.75, 10.5, -7.5, -7.25, -7.0, -6.75, -6.5, -3.5, -3.25, 1.25, 10.25, -7.0, -6.75, -3.5, 9.0, -4.0, -4.25, 17.25, 17.0, 17.0, 3.0, 3.25, 16.5, 16.5, 16.75, 3.0, 13.0, 13.25, 13.5, 13.75, 14.0, 14.25, 14.5, 14.75, 15.0, 15.25, 15.25, 15.5, 15.75, 16.0, 16.25, 16.5, 4.75, 5.0, 10.25, 16.75, 17.0, 17.25, 4.25, 4.5, 4.75, 5.0, 5.25, 5.5, 5.75, 6.0, 6.25, 6.5, 10.25, 4.25, 6.5, 6.75, 7.0, 7.25, 7.5, 7.75, 8.0, 10.0, 10.0]}, {"Y"=[-1.75], "Y"=[8.75]}, {"Y"=[-23.75, -23.5, -23.5, -22.0, -21.75, -17.5, -13.0, -13.0, -12.75, -12.5, -12.25, -11.5, -10.75, -10.75, -10.5, -10.5, -10.5, -10.5, -10.25, -10.25, -10.25, -10.0, -9.75, -9.5, -9.5, -9.5, -9.25, -9.25, -9.0, -9.0, -9.0, -9.0, -8.75, -8.75, -8.75, -8.75, -8.75, -8.75, -8.75, -8.75, -8.75, -8.5, -8.5, -8.5, -8.5, -8.5, -8.5, -8.5, -8.25, -8.25, -8.25, -8.25, -8.25, -8.25, -8.25, -8.25, -8.25, -8.25, -8.25, -8.0, -8.0, -8.0, -8.0, -7.75, -7.75, -7.75, -7.75, -7.75, -7.75, -7.75, -7.75, -7.75, -7.5, -7.5, -7.5, -7.5, -7.5, -7.5, -7.5, -7.5, -7.5, -7.5, -7.5, -7.5, -7.25, -7.25, -7.25, -7.25, -7.25, -7.25, -7.25, -7.25, -7.25, -7.25, -7.25, -7.25, -7.25, -7.25, -7.0, -7.0, -7.0, -7.0, -7.0, -7.0, -7.0, -7.0, -7.0, -7.0, -6.75, -6.75, -6.75, -6.75, -6.75, -6.75, -6.75, -6.75, -6.75, -6.75, -6.75, -6.5, -6.5, -6.5, -6.5, -6.5, -6.25, -6.25, -6.25, -6.25, -6.25, -6.25, -6.25, -6.25, -6.25, -6.25, -6.25, -6.25, -6.0, -6.0, -5.75, -5.75, -5.75, -5.75, -5.75, -5.75, -5.75, -5.75, -5.75, -5.75, -5.75, -5.75, -5.75, -5.75, -5.75, -2.25, -2.25, -2.25, -2.25, -2.25, -2.25, -2.25, -2.25, -2.25, -2.25, -2.25, -2.25, -2.25, -2.25, -2.25, -2.25, -2.25, -2.25, -2.0, -2.0, -2.0, -2.0, -2.0, -2.0, -2.0, -2.0, -2.0, -2.0, -2.0, -2.0, -2.0, -2.0, -2.0, -2.0, -2.0, -2.0, -2.0, -2.0, -2.0, -2.0, -2.0, -2.0, -1.75, -1.75, -1.75, -1.75, -1.75, -1.75, -1.75, -1.75, -1.75, -1.75, -1.75, -1.75, -1.75, -1.75, -1.75, -1.75, -1.75, -1.5, -1.5, -1.5, -1.5, -1.5, -1.5, -1.5, -1.5, -1.5, -1.5, -1.5, -1.5, -1.5, -1.25, -1.25, 1.75, 1.75, 1.75, 1.75, 1.75, 1.75, 1.75, 1.75, 1.75, 1.75, 1.75, 1.75, 1.75, 2.0, 2.0, 2.0, 2.0, 2.0, 2.0, 2.0, 2.0, 2.0, 2.0, 2.25, 2.25, 2.5, 2.5, 2.5, 2.5, 2.5, 2.5, 2.75, 2.75, 2.75, 2.75, 2.75, 2.75, 2.75, 2.75, 2.75, 3.0, 3.0, 3.0, 3.0, 3.0, 3.0, 3.0, 3.0, 3.25, 3.25, 3.25, 3.25, 3.25, 3.25, 3.25, 3.25, 3.5, 3.5, 3.5, 3.5, 3.5, 3.75, 4.0, 4.0, 4.0, 4.0, 4.25, 4.25, 4.25, 4.5, 4.5, 4.5, 4.5, 4.75, 4.75, 4.75, 5.0, 5.0, 5.5, 6.5, 7.0, 7.0, 7.25, 7.5, 7.5, 7.75, 7.75, 8.0, 8.25, 8.5, 8.75, 8.75, 10.5, 10.75, 11.0, 11.0, 11.0, 11.0, 11.0, 11.0, 11.25, 11.25, 11.25, 11.25, 11.25, 11.25, 11.25, 11.25, 11.5, 11.5, 11.5, 11.5, 11.5, 11.5, 11.5, 11.5, 11.5, 11.5, 11.5, 11.5, 11.75, 11.75, 11.75, 11.75, 11.75, 12.0, 12.0, 12.0, 12.0, 12.0, 12.0, 12.0, 12.25, 12.25, 12.5, 12.75, 13.5, 13.5, 13.5, 13.5, 13.5, -2.25, -2.25, -1.75], "Y"=[24.75, 24.75, 25.0, 24.75, 24.75, 15.25, 1.0, 4.5, 20.0, 19.75, 0.5, 14.25, 14.25, 14.5, 6.0, 14.5, 14.75, 15.5, 14.75, 15.0, 15.25, 9.5, 3.5, -3.0, 3.0, 3.25, 8.25, 16.75, 0.5, 1.5, 8.25, 12.25, 1.0, 1.25, 1.5, 2.0, 2.25, 6.0, 8.0, 8.5, 12.75, -11.5, -5.75, 1.0, 2.25, 3.0, 9.0, 12.75, -13.25, -11.0, -4.5, -1.25, 3.0, 3.25, 4.0, 6.5, 8.75, 9.0, 9.25, -15.0, 8.75, 9.0, 9.25, -13.5, -8.0, -6.25, -3.0, -2.75, 1.75, 2.0, 2.25, 9.75, -11.5, -4.5, -2.75, -1.0, -0.75, 0.0, 2.0, 2.75, 3.0, 7.0, 7.25, 7.5, -14.25, -11.5, -8.5, -8.0, -4.75, -4.25, -3.25, -3.0, -0.75, 0.25, 0.75, 2.75, 3.0, 7.75, -14.75, -14.5, -11.5, -8.25, -1.5, -1.25, 1.0, 8.0, 8.25, 10.5, -11.75, 0.25, 0.5, 0.75, 1.5, 2.0, 2.25, 2.5, 6.5, 6.75, 8.25, -19.0, 0.25, 0.5, 0.75, 6.25, -5.75, -2.5, -0.25, 0.0, 0.25, 0.5, 0.75, 1.0, 1.25, 1.5, 1.75, 2.0, 5.0, 6.25, -12.25, -10.0, -5.25, -4.25, -4.0, -3.0, -0.75, -0.5, -0.25, 2.0, 2.25, 2.5, 3.75, 4.0, 5.0, -3.25, -3.0, -2.5, -2.25, 3.0, 3.25, 3.5, 3.75, 4.0, 4.25, 4.5, 4.75, 5.0, 5.25, 5.5, 6.0, 6.5, 7.25, -12.75, -10.75, -9.25, -9.0, -8.0, -7.0, -6.25, -5.5, -5.0, -4.5, -4.0, -3.5, -3.25, -3.0, -2.75, -2.5, -2.25, 3.0, 3.25, 3.5, 3.75, 4.25, 4.5, 15.25, -15.5, -12.75, -10.75, 3.5, 3.75, 4.0, 4.25, 4.5, 4.75, 5.0, 5.25, 5.75, 6.25, 6.75, 7.25, 8.0, 15.25, -12.75, -10.75, -9.25, -8.0, -7.0, -6.25, -5.75, -5.25, -5.0, -4.5, -4.25, -3.75, -3.5, -15.75, -12.75, 3.25, 3.5, 3.75, 4.0, 4.25, 4.5, 4.75, 5.0, 5.25, 5.75, 6.25, 6.75, 7.25, -13.0, -4.5, -4.25, -3.75, 6.0, 6.25, 6.75, 7.25, 8.0, 8.75, 3.75, 10.0, 4.25, 4.5, 4.75, 6.0, 7.75, 11.25, -7.0, -6.0, -5.25, 7.5, 7.75, 8.5, 9.5, 9.75, 12.75, -12.5, -12.25, -6.75, -6.0, -5.75, 8.25, 8.5, 9.25, -10.5, -8.75, -8.5, 9.0, 10.25, 10.5, 12.5, 15.25, -15.5, -15.0, -10.5, -8.75, 10.5, -3.25, -12.5, -12.25, -10.0, -6.25, -8.0, -5.5, 2.25, -9.75, -8.0, -6.25, -4.75, -12.75, -5.25, -5.0, -12.5, 1.5, 1.5, 3.75, 1.25, 5.5, 5.5, 3.5, 5.75, 1.75, 3.5, 3.5, 8.0, 3.75, -1.5, 8.25, 3.5, 3.0, 2.5, 4.0, 4.25, 4.75, 5.25, 9.25, -5.5, -3.75, -2.0, 1.75, 3.25, 3.5, 8.5, 10.75, -7.5, -5.25, 1.25, 3.0, 3.25, 3.5, 8.0, 8.5, 9.5, 9.75, 10.25, 10.5, -7.5, -5.25, 1.75, 2.0, 7.5, -4.5, -4.25, -3.75, 6.75, 8.0, 13.75, 14.0, -3.5, 13.5, 12.25, 12.5, -0.75, -0.5, -0.25, 0.0, 0.25, 8.75, 12.75, 8.75]}, {"Y"=[0.85, 0.95, 0.95, 0.6, 0.6, 0.85, 0.85, -0.85, -0.85, -0.95, -0.95, -0.6, -0.6, -0.85, -0.6, -0.6, -0.85, -0.85, 0.85, 0.85], "Y"=[-0.6, -0.6, -1.4, -1.4, -0.6, -0.6, 2.4, 2.4, -0.6, -0.6, -1.4, -1.4, -0.6, -0.6, -0.6, -1.4, -1.4, -1.6, -1.6, -1.4]}]
  in  "Make WPT":bool
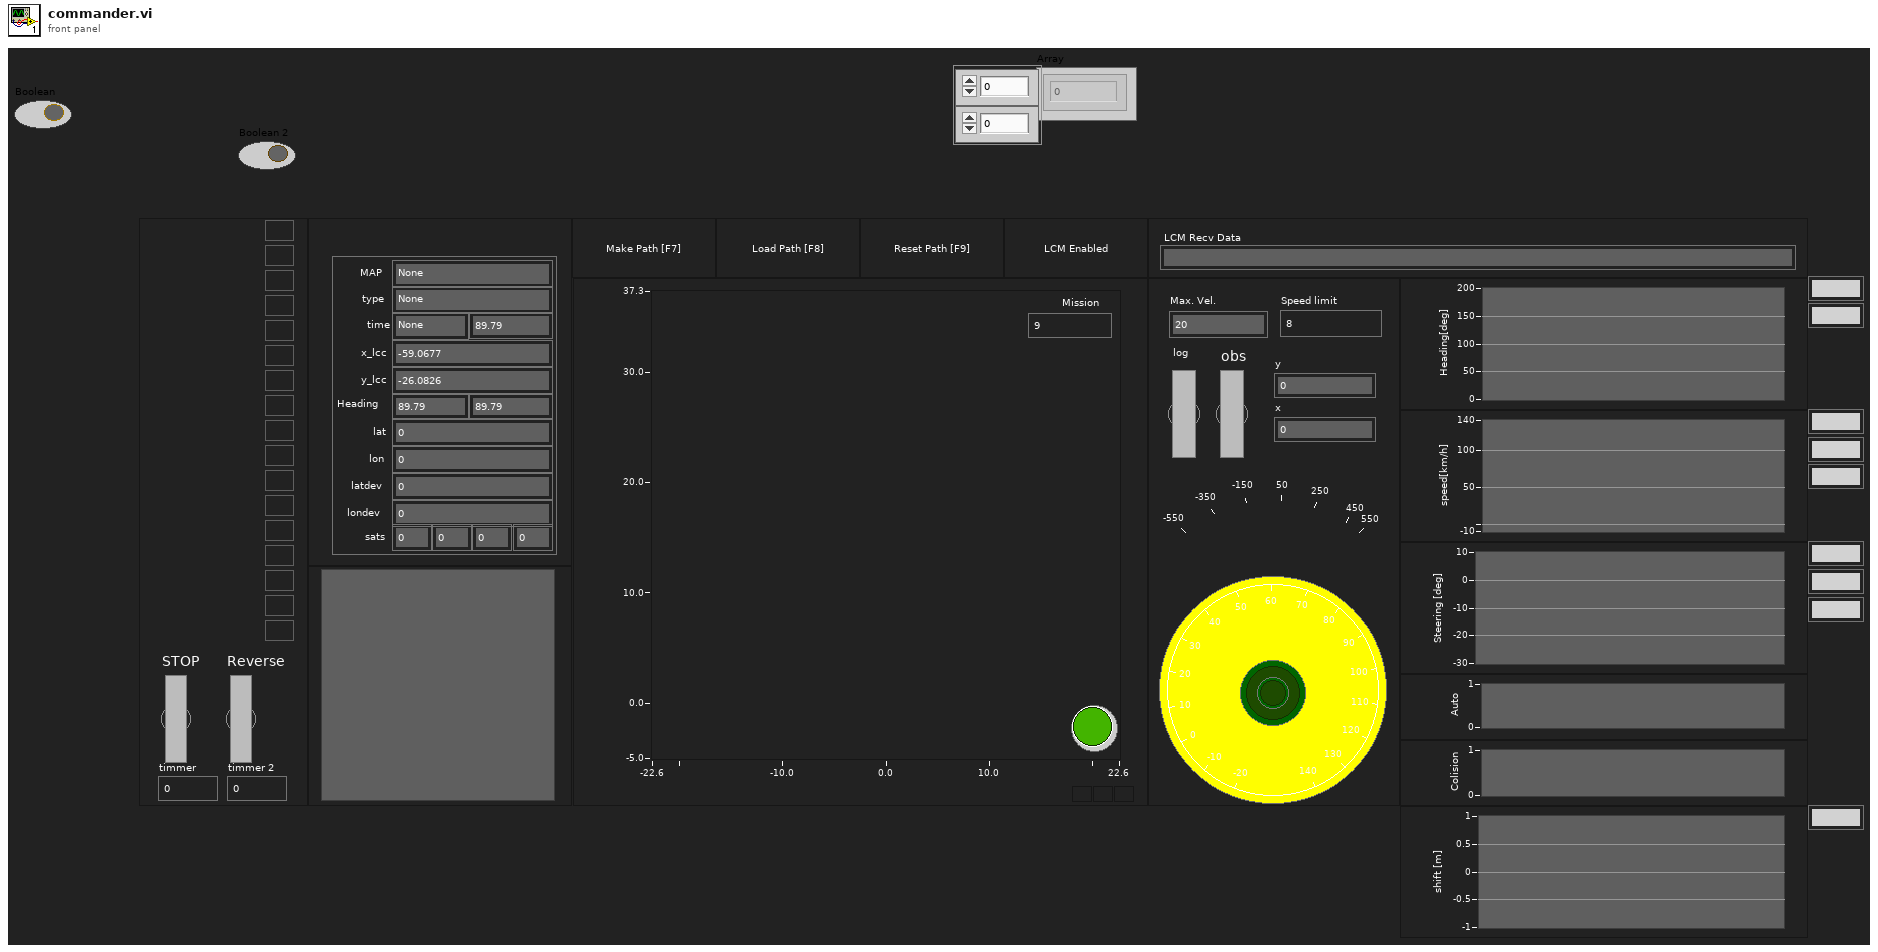
[diagram p1: front panel]
types:
  T1 = cluster{"type":string, "x_lcc":dbl, "y_lcc":dbl, "latdev":sgl, "londev":sgl, "sats":u8, "gps_l1_ranges":u8, "gps_l1_mask_ranges":u8, "gps_l2_mask_ranges":u8, "Heading":dbl, "lon":sgl, "lat":sgl, "time":string, "hgps":dbl, "lag":dbl, "MAP":string}
  T2 = cluster{"Steer_input":dbl, "Steer_output":dbl, "handle":dbl}
  T3 = cluster{"VS_des":dbl, "VS_can":dbl, "VS_des":dbl}
  T4 = cluster{"X":cluster{"idx":i32, "x":dbl, "y":dbl, "h":dbl, "x_path":dbl}}[]
  T5 = cluster{"idx":i32, "x":dbl, "y":dbl, "h":dbl, "x_path":dbl}
  T6 = cluster{"idx":i32, "x":dbl, "y":dbl, "hp":dbl, "x_path":dbl}
  T7 = cluster{"GPSTime":dbl, "attitude[2]":dbl, "lcc[0]":dbl, "lcc[1]":dbl, "heading_GPS":dbl}
  T8 = cluster{"Steer_input":dbl, "Steer_output":dbl, "VS_des":dbl, "VS_can":dbl, "heading":dbl, "auto":bool, "run":bool, "x":dbl, "y":dbl}
  T9 = cluster{"c_idx":i32, "xc":dbl, "yc":dbl, "hc":dbl, "xc_path":dbl}
  T10 = cluster{"Minimum":dbl, "Minimum":dbl, "Minimum":dbl, "Minimum":dbl, "Minimum":dbl}
  T11 = cluster{"X":cluster{"c_idx":i32, "xc":dbl, "yc":dbl, "hc":dbl, "xc_path":dbl}}[]
  T12 = cluster{"x":cluster{"idx":i32, "x":dbl, "y":dbl, "h":dbl, "x_path":dbl}}[]
  T13 = cluster{"hash":i64, "sys time":i64, "time":dbl, "x":dbl, "y":dbl, "h":dbl, "numSV":i32, "postype":i32, "lag":i32, "hordev":dbl, "lat":dbl, "lon":dbl, "hgt":dbl, "map_idx":i32}
  T14 = typedef "NI_Matrix.lvlib/RealMatrix.ctl" = dbl[][]
  T15 = cluster{"hash":i64, "sys time":i64, "dt":dbl, "x":dbl, "y":dbl, "speed":dbl, "heading":dbl, "yaw_rate":dbl}
  T16 = cluster{"hash":i64, "sys time":i64, "time":dbl, "yaw_rate":dbl, "mdps torque":dbl, "mdps str_ang":dbl, "VS_CAN":dbl, "lat_accel":dbl, "mcp":dbl, "accel pedal value":dbl, "tps":dbl, "odometer":dbl, "battery voltage":dbl, "WHL_SPD_RR":dbl, "WHL_SPD_RL":dbl, "WHL_SPD_FR":dbl, "WHL_SPD_FL":dbl}
  T17 = cluster{"hash":dbl, "sys time":dbl, "dt":dbl, "x":dbl, "y":dbl, "speed":dbl, "heading":dbl, "yaw_rate":dbl}
  T18 = cluster{"idx":bool, "x":bool, "y":bool, "h":bool, "x_path":bool}
  T19 = cluster{"idx":dbl, "x":dbl, "y":dbl, "h":dbl, "x_path":dbl}
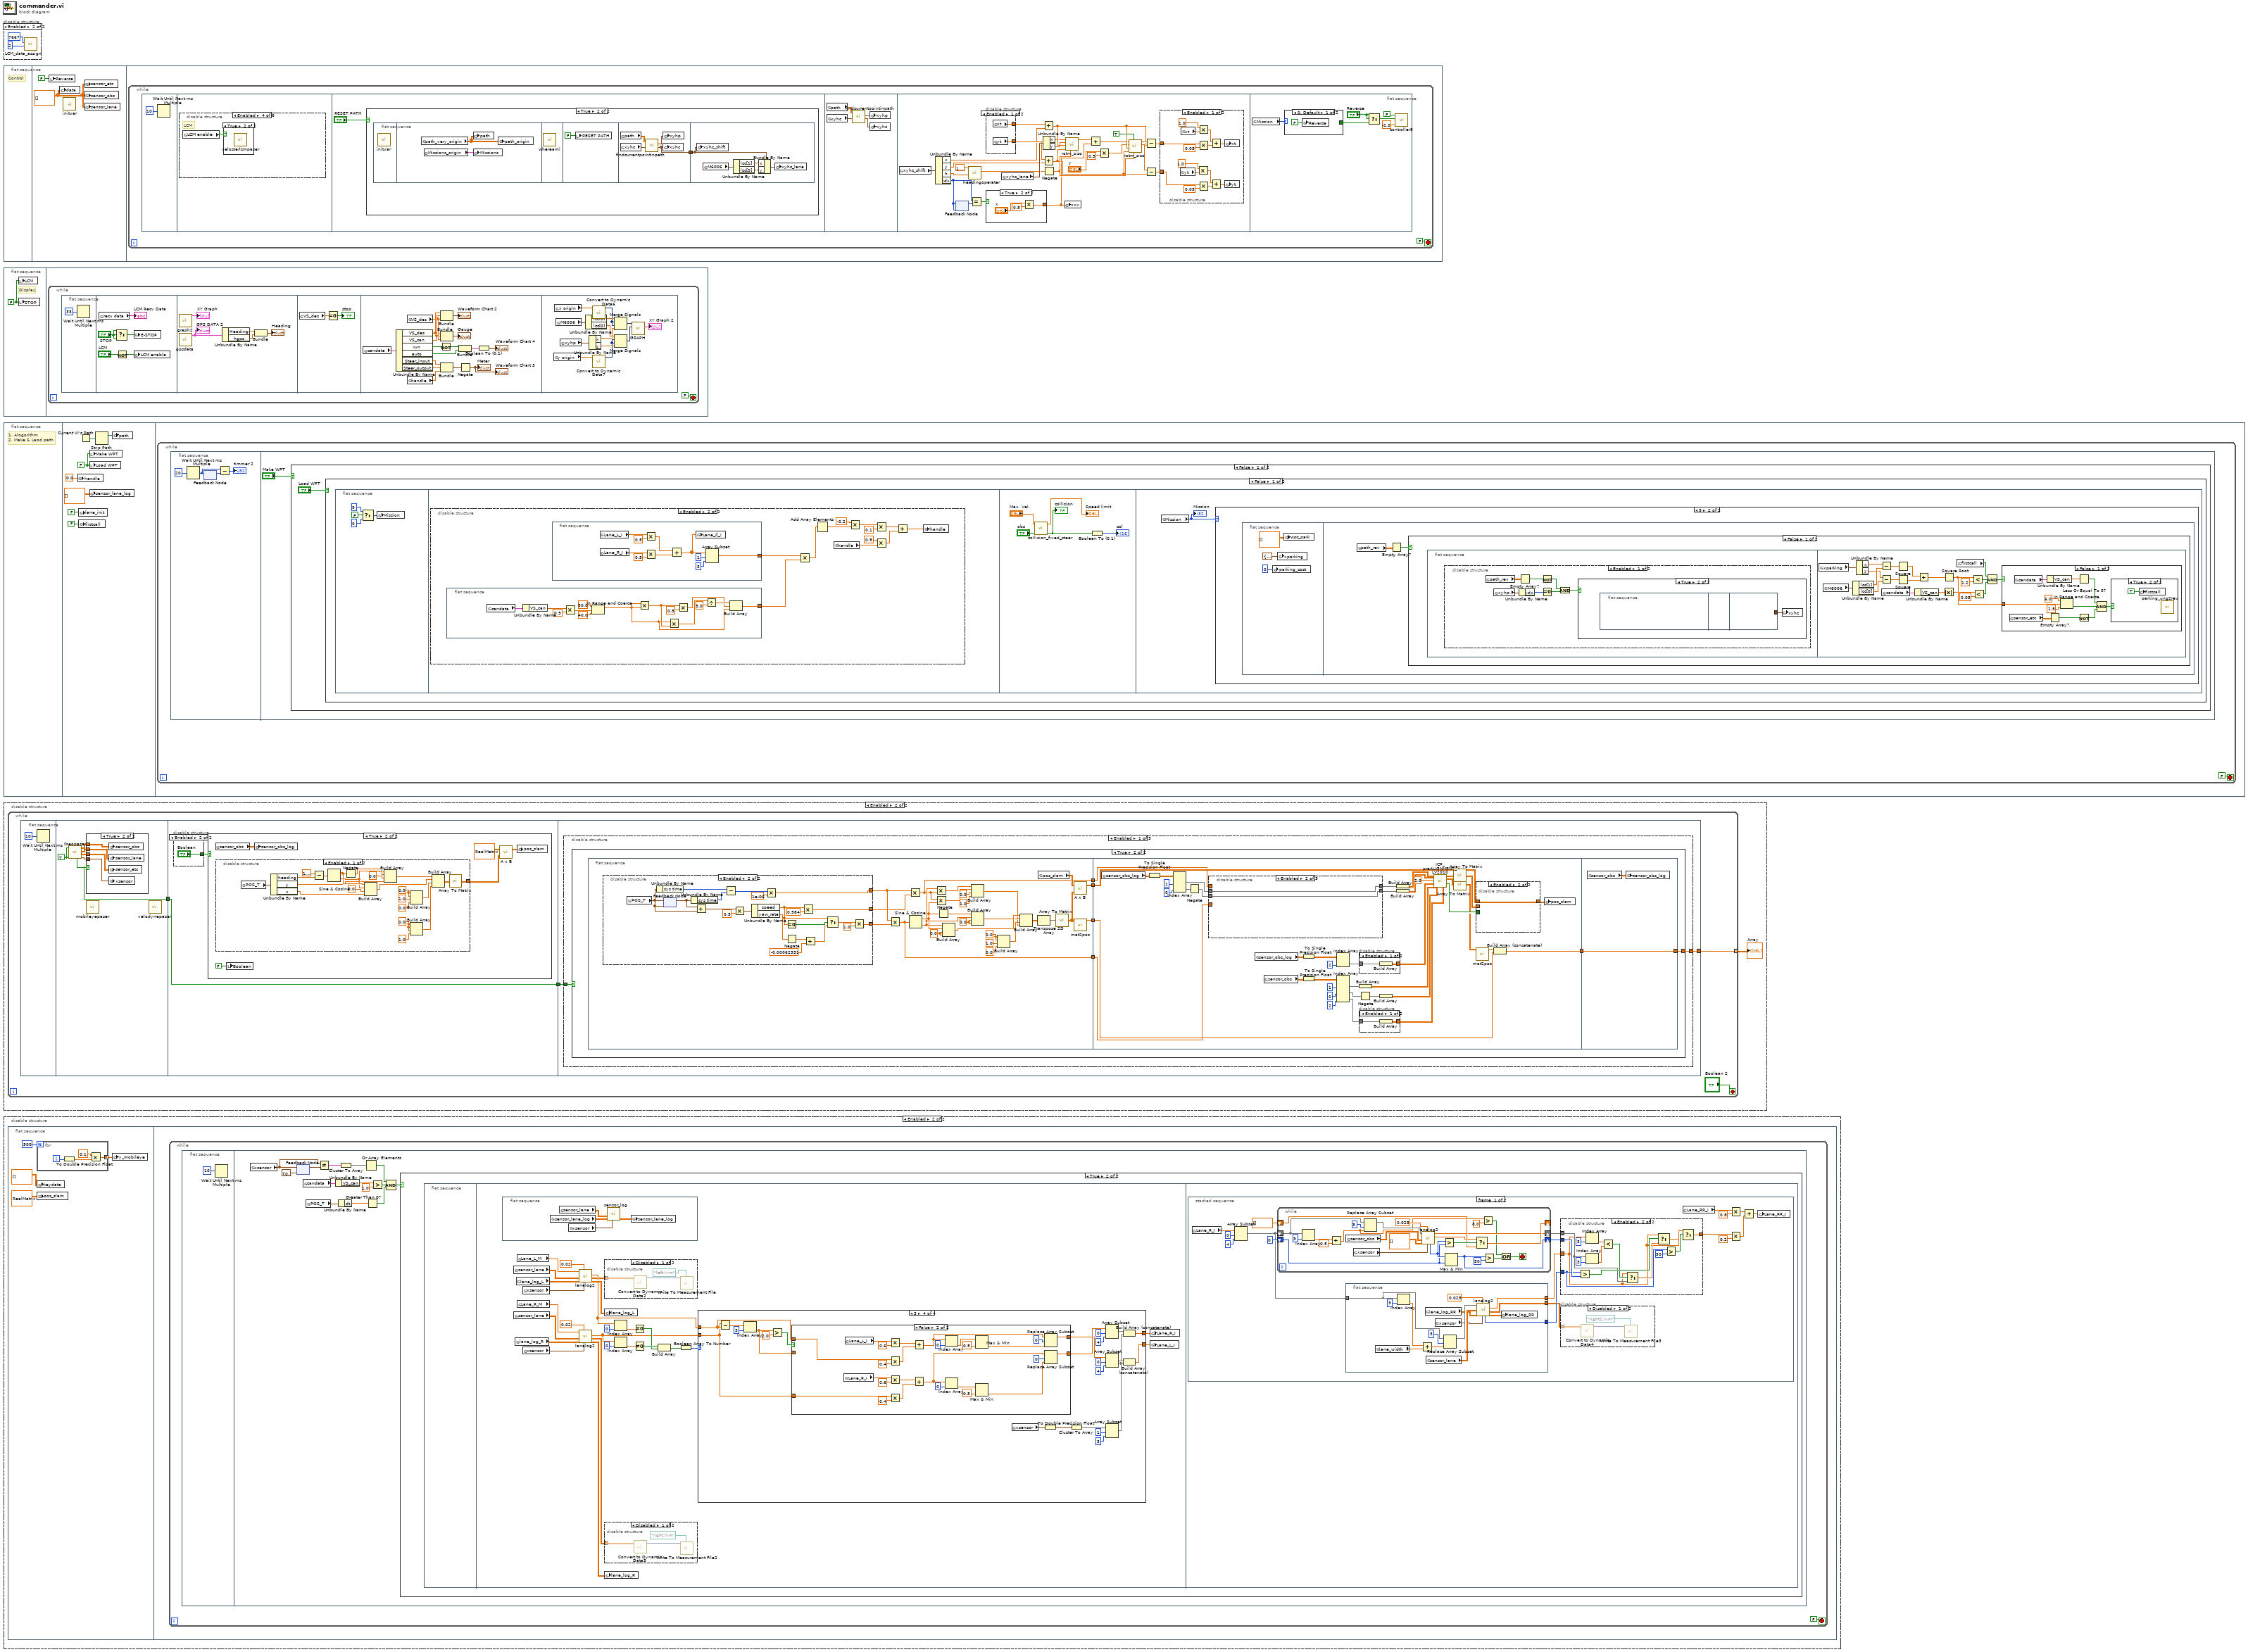
[diagram p0: block diagram]
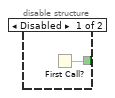
[diagram p4: hidden frame]
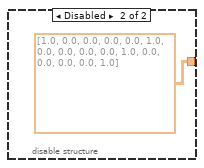
[diagram p6: hidden frame]
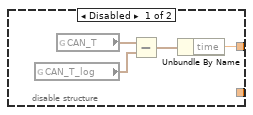
[diagram p8: hidden frame]
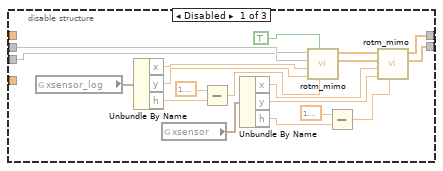
[diagram p11: hidden frame]
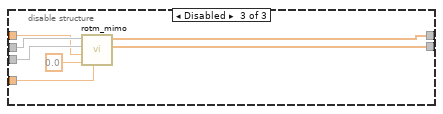
[diagram p12: hidden frame]
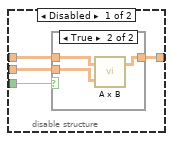
[diagram p13: hidden frame]
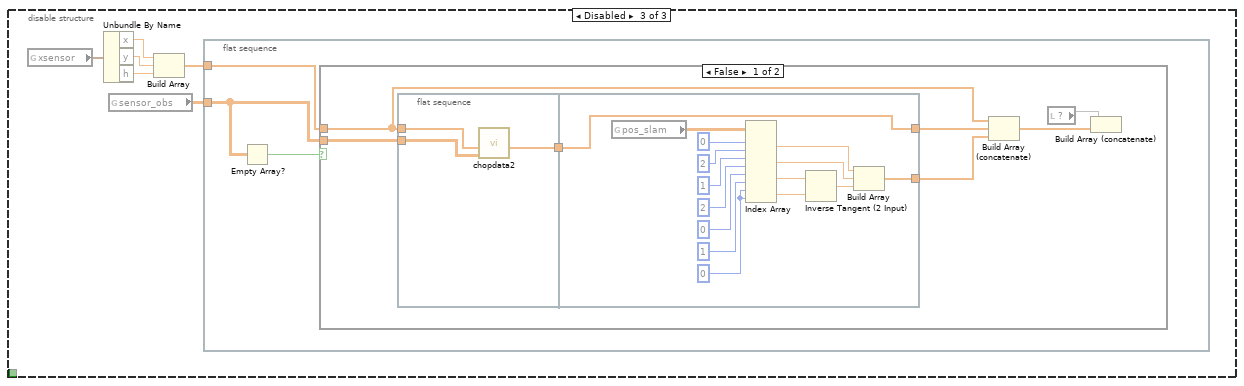
[diagram p16: hidden frame]
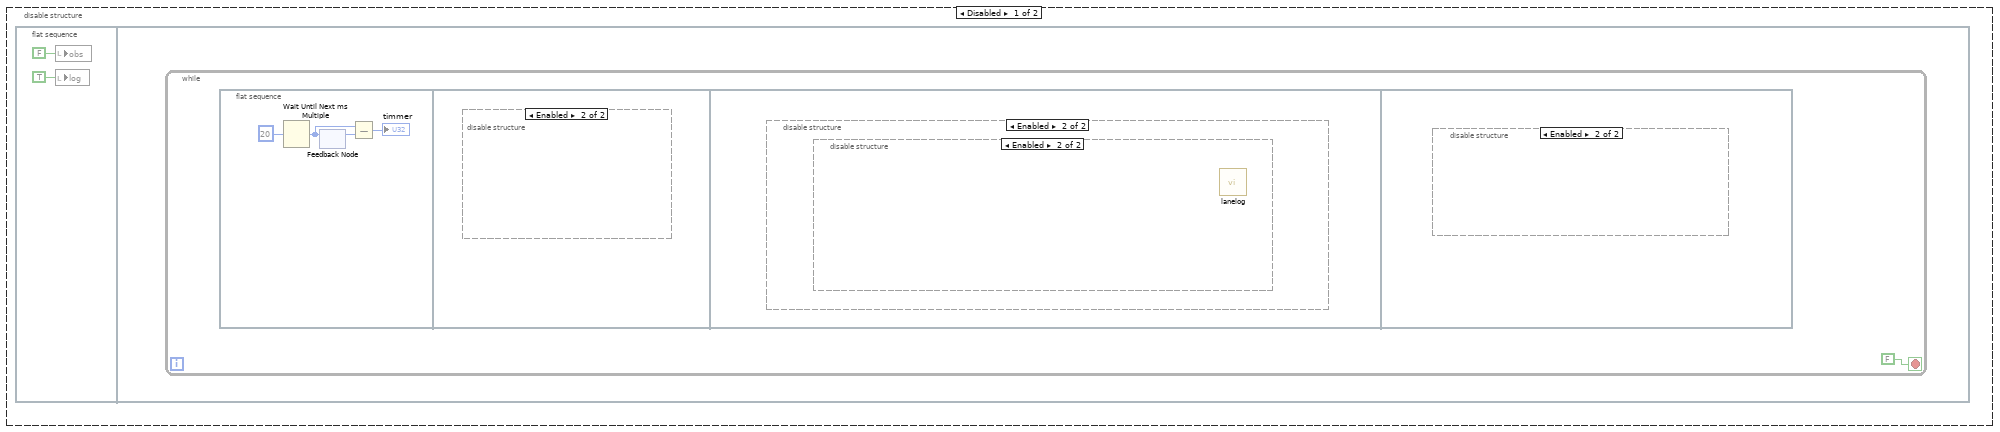
[diagram p18: hidden frame]
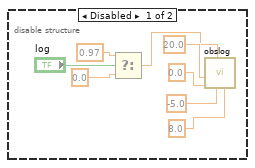
[diagram p19: hidden frame]
diagram:
  n1 = disable-structure shown="Enabled" {
    frame Disabled {
      n2 = call "comm.vi"() -> ()  [unwired: 12 in]
    }
    frame Enabled {
      n3 = call "LCM_data_assign.vi"("time-to-live"=u16 2, "port"=u16 7667) -> ()  [unwired: 10 in]
    }
  }
  n4 = flat-sequence {
    frame #0 {
      # "Control"
    }
    frame #1 {
      w3 = dbl[][] [] ("sensor_car")
      n5 = local write "Reverse"(FALSE ("STOP Signal")) -> ()
      n6 = global write "G_SEN.vi" "data"(w3) -> ()
      n7 = call "initvar.vi"() -> ()  [unwired: 12 in]
      n8 = global write "G_SEN.vi" "sensor_etc"(w3) -> ()
      n9 = global write "G_SEN.vi" "sensor_obs"(w3) -> ()
      n10 = global write "G_SEN.vi" "sensor_lane"(w3) -> ()
    }
    frame #2 {
      n11 = while {
        stop <- FALSE ("Boolean") stop-if-true
        n12 = flat-sequence {
          frame #0 {
            n13 = Wait Until Next ms Multiple(millisecond multiple=u32 10 ("milliseconds to wait")) -> ()  [unwired: 1 out]
          }
          frame #1 {
            n14 = disable-structure shown="Enabled" {
              frame Disabled {
                n15 = global read "G_DATA.vi" "Load data"() -> (w7:bool)
                n16 = case shown="False" w7 {
                  frame False {
                    # "soul"
                    n17 = call "soulpaser.vi"("rionav?"=FALSE) -> ()  [unwired: 11 in]
                  }
                  frame True {
                  }
                }
              }
              frame Disabled {
                n18 = global read "G_DATA.vi" "Load data"() -> (w9:bool)
                n19 = case shown="False" w9 {
                  frame False {
                    # "veloster"
                    n20 = call "velosterpaser.vi"("x"=0.0) -> ()  [unwired: 11 in]
                  }
                  frame True {
                  }
                }
              }
              frame Disabled {
                n21 = global read "G_DATA.vi" "Load data"() -> (w11:bool)
                n22 = case shown="True" w11 {
                  frame False {
                    # "webot"
                    n23 = call "webot.vi"() -> ()  [unwired: 12 in]
                  }
                  frame True {
                  }
                }
              }
              frame Enabled {
                # "LCM"
                n24 = global read "G_LCM.vi" "LCM enable"() -> (w12:bool)
                n25 = case shown="True" w12 {
                  frame False {
                  }
                  frame True {
                    n26 = call "velosterlcmpaser.vi"() -> ()  [unwired: 12 in]
                  }
                }
              }
              frame Disabled {
              }
              frame Disabled {
                # "RCcar"
                n27 = global read "G_DATA.vi" "Load data"() -> (w13:bool)
                n28 = case shown="True" w13 {
                  frame False {
                  }
                  frame True {
                    n29 = global read "G_VEH.vi" "VS_des"() -> (w14:dbl)
                    n30 = global read "G_VEH.vi" "handle"() -> (w15:dbl)
                    n31 = shared-variable "NI-sbRIO9606-01866155\\sharedvari.lvlib\\vs_des"(w14) -> ()  [unwired: 1 in, 1 out]
                    n32 = shared-variable "NI-sbRIO9606-01866155\\sharedvari.lvlib\\steer_input"(w15) -> ()  [unwired: 1 in, 1 out]
                  }
                }
              }
            }
          }
          frame #2 {
            n33 = case shown="True" "RESET PATH" {
              frame False {
                n34 = disable-structure shown="Enabled" {
                  frame Enabled {
                  }
                  frame Disabled {
                    n35 = call "commpaser.vi"("y_shift"=1.7000000000000006, "large map"=TRUE) -> ("lane"=w23:dbl[][], "obs"=w24:dbl[][], "size(s)"=w28:i32, "etc"=w21:dbl[][])  [unwired: 5 in, 1 out]
                    n36 = call "Ibeopaser.vi"() -> ("etc"=w17:dbl[][], "lane"=w18:dbl[][], "obs"=w19:dbl[][])  [unwired: 7 in, 2 out]
                    n37 = disable-structure shown="Disabled" {
                      disable-tunnel: [w31 w34 w42] -> w25
                      disable-tunnel: w19 -> [w31 _ w41]
                      disable-tunnel: w24 -> [_ w34 w40]
                      disable-tunnel: w23 -> [_ w33 w39]
                      disable-tunnel: w18 -> [w30 _ w38]
                      disable-tunnel: [w30 w33 w37] -> w22
                      disable-tunnel: w21 -> [_ w32 w36]
                      disable-tunnel: [w29 w32 w35] -> w20
                      disable-tunnel: w17 -> [w29 _ _]
                      frame Enabled {
                        # "ibeo"
                      }
                      frame Disabled {
                        # "velodyne"
                      }
                      frame Disabled {
                        # "both"
                        n38 = Build Array (concatenate)(w41, w40) -> (w42:dbl[][])
                        n39 = Build Array (concatenate)(w38, w39) -> (w37:dbl[][])
                        n40 = Build Array (concatenate)(w36) -> (w35:dbl[][])  [unwired: 1 in]
                      }
                    }
                    n41 = global write "G_SEN.vi" "sensor_obs"(w25) -> ()
                    n42 = global write "G_SEN.vi" "sensor_lane"(w22) -> ()
                    n43 = global write "G_SEN.vi" "sensor_etc"(w20) -> ()
                  }
                }
              }
              frame True {
                n44 = flat-sequence {
                  tunnel: [w48] -> w43
                  tunnel: w43 -> [w55]
                  frame #0 {
                    n45 = call "initvar.vi"() -> ()  [unwired: 12 in]
                  }
                  frame #1 {
                    n46 = global read "G_PATH.vi" "path_very_origin"() -> (w45:dbl[][])
                    n47 = global read "G_PATH.vi" "Missions_origin"() -> (w44:T4)
                    n48 = global write "G_PATH.vi" "path"(w45) -> ()
                    n49 = global write "G_PATH.vi" "Missions"(w44) -> ()
                    n50 = global write "G_PATH.vi" "path_origin"(w45) -> ()
                  }
                  frame #2 {
                    n51 = call "whereami.vi"() -> ()  [unwired: 12 in]
                  }
                  frame #3 {
                    n52 = local write "RESET PATH"(FALSE ("RESET PATH")) -> ()
                  }
                  frame #4 {
                    n53 = global read "G_PATH.vi" "path"() -> (w47:dbl[][])
                    n54 = global read "G_VEH.vi" "xyhc"() -> (w49:T5)
                    n55 = call "findcurrentpointinpath.vi"("xyhc_in"=w49, "path_updated"=w47) -> ("xyhc_out"=w48:T5, "xyhp"=w50:T6)  [unwired: 8 in]
                    n56 = global write "G_VEH.vi" "xyhp"(w50) -> ()
                    n57 = global write "G_VEH.vi" "xyhc"(w48) -> ()
                  }
                  frame #5 {
                    n58 = global write "G_VEH.vi" "xyhc_shift"(w55) -> ()
                    n59 = global read "G_NAV.vi" "M6006"() -> (w53:T7)
                    n60 = Unbundle By Name(w53) -> ("lcc[1]"=w52:dbl, "lcc[0]"=w51:dbl)
                    n61 = Bundle By Name(cluster=w55, "x"=w52, "y"=w51) -> (w54:T5)
                    n62 = global write "G_VEH.vi" "xyhc_lane"(w54) -> ()
                  }
                }
              }
            }
          }
          frame #3 {
            n63 = global read "G_PATH.vi" "path"() -> (w56:dbl[][])
            n64 = global read "G_VEH.vi" "xyhc"() -> (w59:T5)
            n65 = call "findcurrentpointinpath.vi"("xyhc_in"=w59, "path_updated"=w56) -> ("xyhc_out"=w57:T5, "xyhp"=w58:T6)  [unwired: 8 in]
            n66 = global write "G_VEH.vi" "xyhp"(w58) -> ()
            n67 = global write "G_VEH.vi" "xyhc"(w57) -> ()
          }
          frame #4 {
            n68 = global read "G_VEH.vi" "xyhc_shift"() -> (w69:T5)
            n69 = Unbundle By Name(w69) -> ("x"=w72:dbl, "y"=w74:dbl, "h"=w78:dbl, "idx"=w66:i32)
            n70 = feedback-in #1(w66) -> ()
            n71 = feedback #1(w66) -> (w67:i32)
            n72 = call "headingoperater.vi"("h1"=w78, "h2"=1.5707963267948966) -> ("h2-h1"=w85:dbl)  [unwired: 8 in, 1 out]
            n73 = Equal?(x=w66, y=w67) -> (x = y?=w65:bool)
            n74 = disable-structure shown="Enabled" {
              disable-tunnel: [w107 _] -> w73
              disable-tunnel: [w106 _] -> w75
              frame Enabled {
                n75 = global read "G_PATH.vi" "xt"() -> (w107:dbl)
                n76 = global read "G_PATH.vi" "yt"() -> (w106:dbl)
              }
              frame Disabled {
              }
            }
            n77 = case shown="True" w65 {
              tunnel: [w88 w90] -> w61
              frame False {
                w88 = 0.0 ("x")
                n78 = local write "x"(w88) -> ()
              }
              frame True {
                n79 = Multiply(x="x", y=0.5) -> (x*y=w90:dbl)
              }
            }
            n80 = global read "G_VEH.vi" "xyhc_lane"() -> (w87:T5)
            n81 = Add(x=w73, y=w72) -> (x+y=w80:dbl)
            n82 = Add(x=w75, y=w74) -> (x+y=w81:dbl)
            n83 = Negate(x=w85) -> (-x=w86:dbl)
            n84 = Unbundle By Name(w87) -> ("x"=w71:dbl, "y"=w70:dbl)
            n85 = global write "G_PATH.vi" "xxx"(w61) -> ()
            n86 = call "rotm_siso.vi"("angle[rad]"=w86, "y0"=w81, "x0"=w80, "y"=w70, "x"=w71) -> ("x'"=w62:dbl)  [unwired: 5 in, 1 out]
            n87 = Add(x=w62, y=w61) -> (x+y=w68:dbl)
            n88 = Multiply(x="y", y=0.5) -> (x*y=w63:dbl)
            n89 = call "rotm_siso.vi"("angle[rad]"=w86, "reverse"=TRUE, "y0"=w81, "x0"=w80, "y"=w63, "x"=w68) -> ("y'"=w84:dbl, "x'"=w83:dbl)  [unwired: 4 in]
            n90 = Subtract(x=w83, y=w80) -> (x-y=w76:dbl)
            n91 = Subtract(x=w84, y=w81) -> (x-y=w77:dbl)
            n92 = disable-structure shown="Enabled" {
              disable-tunnel: w76 -> [w99 _]
              disable-tunnel: w77 -> [w93 _]
              frame Enabled {
                n93 = global read "G_PATH.vi" "yt"() -> (w96:dbl)
                n94 = global read "G_PATH.vi" "xt"() -> (w103:dbl)
                n95 = Multiply(x=1.0, y=w96) -> (x*y=w95:dbl)
                n96 = Multiply(x=1.0, y=w103) -> (x*y=w101:dbl)
                n97 = Multiply(x=w99, y=0.05 ("x")) -> (x*y=w98:dbl)
                n98 = Multiply(x=w93, y=0.05 ("x")) -> (x*y=w92:dbl)
                n99 = Add(x=w101, y=w98) -> (x+y=w105:dbl)
                n100 = Add(x=w95, y=w92) -> (x+y=w104:dbl)
                n101 = global write "G_PATH.vi" "xt"(w105) -> ()
                n102 = global write "G_PATH.vi" "yt"(w104) -> ()
              }
              frame Disabled {
              }
            }
          }
          frame #5 {
            n103 = global read "G_PATH.vi" "Mission"() -> (w108:i32)
            n104 = case shown="0, Default" w108 {
              tunnel: [_ w115] -> w112
              frame 0, Default {
                n105 = global write "G_VEH.vi" "Reverse"(FALSE ("Reverse")) -> ()
              }
              frame 9 {
                n106 = global read "G_VEH.vi" "Reverse"() -> (w115:bool)
              }
            }
            n107 = Select(t="Reverse", s="Reverse", f=w112) -> (s? t:f=w111:bool)
            n108 = call "controller8.vi"("Neg max speed"=-2.0, "reverse"=w111, "slowmode"=FALSE ("slow mode")) -> ()  [unwired: 9 in]
          }
        }
      }
    }
  }
  n109 = flat-sequence {
    frame #0 {
      w116 = FALSE ("LCM")
      # "Display"
      n110 = local write "LCM"(w116) -> ()
      n111 = local write "STOP"(w116) -> ()
    }
    frame #1 {
      n112 = while {
        stop <- FALSE ("exit") stop-if-true
        n113 = flat-sequence {
          frame #0 {
            n114 = Wait Until Next ms Multiple(millisecond multiple=u32 33 ("milliseconds to wait")) -> ()  [unwired: 1 out]
          }
          frame #1 {
            n115 = global read "G_LCM.vi" "recv data"() -> (→"LCM Recv Data":string)
            n116 = Select(t="STOP", s="STOP", f="STOP") -> (s? t:f=w123:bool)
            n117 = Not(x="LCM") -> (.not. x?=w120:bool)
            n118 = global write "G_VEH.vi" "E-STOP"(w123) -> ()
            n119 = global write "G_LCM.vi" "LCM enable"(w120) -> ()
          }
          frame #2 {
            n120 = call "graph2.vi"() -> ("XY Graph"=→"XY Graph":cluster{"Y":dbl[], "Y":dbl[]}[])  [unwired: 10 in, 1 out]
            n121 = call "gpsdata.vi"() -> ("GPS DATA 2"=w126:T1)  [unwired: 11 in]
            "GPS DATA 2" <- w126
            n122 = Unbundle By Name(w126) -> ("Heading"=w128:dbl, "hgps"=w127:dbl)
            n123 = Bundle("Heading"=w128, "hgps"=w127) -> (→"Heading":cluster{"Heading":dbl, "hgps":dbl})  [unwired: 1 in]
          }
          frame #3 {
            n124 = global read "G_VEH.vi" "VS_des"() -> (w130:dbl)
            n125 = Equal To 0?(x=w130) -> (x = 0?=→"stop":bool)
          }
          frame #4 {
            n126 = global read "G_VEH.vi" "candata"() -> (w146:T8)
            n127 = Unbundle By Name(w146) -> ("VS_des"=w138:dbl, "VS_can"=w139:dbl, "run"=w133:bool, "auto"=w134:bool, "Steer_input"=w132:dbl, "Steer_output"=w131:dbl)
            n128 = global read "G_VEH.vi" "VS_des"() -> (w137:dbl)
            n129 = global read "G_VEH.vi" "handle"() -> (w135:dbl)
            n130 = Not(x=w133) -> (.not. x?=w141:bool)
            n131 = Bundle("VS_des"=w138, "VS_can"=w139, "VS_des"=w137) -> (→"Waveform Chart 2":T3)  [unwired: 1 in]
            n132 = Bundle("VS_des"=w138, "VS_can"=w139, "VS_des"=w137) -> (→"Gauge":T3)  [unwired: 1 in]
            n133 = Bundle("Steer_input"=w132, "Steer_output"=w131, "handle"=w135) -> (w145:T2)  [unwired: 1 in]
            n134 = Bundle(w141, "auto"=w134) -> (w143:cluster{bool, "auto":bool})  [unwired: 1 in]
            n135 = Negate(x=w145) -> (-x=→"Meter" →"Waveform Chart 3":T2)
            n136 = Boolean To (0,1)(Boolean=w143) -> (0, 1=→"Waveform Chart 4":cluster{i16, "auto":i16})
          }
          frame #5 {
            n137 = global read "G_PATH.vi" "y origin"() -> (w148:dbl[])
            n138 = global read "G_PATH.vi" "x origin"() -> (w149:dbl[])
            n139 = global read "G_NAV.vi" "M6006"() -> (w155:T7)
            n140 = global read "G_VEH.vi" "xyhp"() -> (w147:T5)
            n141 = Unbundle By Name(w155) -> ("lcc[1]"=w156:dbl, "lcc[0]"=w157:dbl)
            n142 = Unbundle By Name(w147) -> ("x"=w151:dbl, "y"=w150:dbl)
            n143 = call "Convert to Dynamic Data6"("Array"=w149) -> ("Dynamic Data Type"=w159:dynamicdata)  [unwired: 3 in]
            n144 = call "Convert to Dynamic Data7"("Array"=w148) -> ("Dynamic Data Type"=w158:dynamicdata)  [unwired: 3 in]
            n145 = Merge Signals(w156, w159, w159, w151) -> (w153:dynamicdata)
            n146 = Merge Signals(w157, w158, w158, w150) -> (w154:dynamicdata)
            n147 = call "GRAPH"("Y Input"=w154, "X Input"=w153) -> ("XY Graph"=→"XY Graph 2":cluster{"Y":dbl[], "Y":dbl[]}[])  [unwired: 3 in, 6 out]
          }
        }
      }
    }
  }
  n148 = flat-sequence {
    frame #0 {
      # "1. Alogorithm\n2. Make & Laod path"
    }
    frame #1 {
      w166 = FALSE ("Make WPT")
      n149 = global write "G_VEH.vi" "handle"(0.0 ("handle")) -> ()
      n150 = global write "G_PATH.vi" "lane_init"(FALSE ("lane_init")) -> ()
      n151 = global write "G_VEH.vi" "firstcall"(FALSE ("firstcall")) -> ()
      n152 = Current VI's Path() -> (path=w162:path)
      n153 = local write "Make WPT"(w166) -> ()
      n154 = local write "Load WPT"(w166) -> ()
      n155 = global write "G_SEN.vi" "sensor_lane_log"(dbl[][] [] ("sensor_lane_log")) -> ()
      n156 = Strip Path(path=w162) -> (stripped path=w161:path)  [unwired: 1 out]
      n157 = global write "G_DATA.vi" "path"(w161) -> ()
    }
    frame #2 {
      n158 = while {
        stop <- FALSE stop-if-true
        n159 = flat-sequence {
          frame #0 {
            n160 = Wait Until Next ms Multiple(millisecond multiple=u32 20 ("milliseconds to wait")) -> (millisecond timer value=w168:u32)
            n161 = feedback #2() -> (w170:u32)  [unwired: 1 in]
            n162 = feedback-in #2(w168) -> ()
            n163 = Subtract(x=w168, y=w170) -> (x-y=→"timmer 2":u32)
          }
          frame #1 {
            n164 = case shown="False" "Make WPT" {
              frame False {
                n165 = case shown="False" "Load WPT" {
                  frame False {
                    n166 = flat-sequence {
                      frame #0 {
                        n167 = Select(t=9 ("Mission"), s=FALSE ("Parking mode"), f=0 ("Mission")) -> (s? t:f=w174:i32)
                        n168 = global write "G_PATH.vi" "Mission"(w174) -> ()
                      }
                      frame #1 {
                        n169 = disable-structure shown="Enabled" {
                          frame Disabled {
                            n170 = global read "G_PATH.vi" "lane_width"() -> (w209:dbl)
                            n171 = Multiply(x=w209, y=0.5) -> (x*y=w204:dbl)
                            n172 = global read "G_VEH.vi" "theta handle"() -> (w211)
                            n173 = Add(x=w204, y=0.25) -> (x+y=w202:dbl)
                            n174 = Decrement(x=w202) -> (x-1=w198:dbl)
                            n175 = Multiply(x=0.75, y=w211) -> (x*y=w215:dbl)
                            n176 = Multiply(x=w198, y=10.0) -> (x*y=w196:dbl)
                            n177 = Max & Min(x=0.0, y=w196) -> (max(x,y)=w206:dbl)  [unwired: 1 out]
                            n178 = Negate(x=w206) -> (-x=w205:dbl)
                            n179 = feedback #3() -> (w195:dbl)  [unwired: 1 in]
                            "Waveform Chart 5" <- w195
                            n180 = call "findmovablepath.vi"("x"=w195) -> ("shift"=w189:dbl, "theta handle"=w185:dbl)  [unwired: 9 in]
                            n181 = disable-structure shown="Disabled" {
                              disable-tunnel: w185 -> [w217 w218]
                              disable-tunnel: [w216 w218] -> w184
                              frame Disabled {
                                n182 = feedback #4(w217) -> (w216:dbl)
                                n183 = feedback-in #4(w217) -> ()
                              }
                              frame Enabled {
                              }
                            }
                            n184 = Equal To 0?(x=w189) -> (x = 0?=→"x = 0?":bool)
                            n185 = Sign(1:w189) -> (0:w193:dbl)
                            n186 = Sign(1:w195) -> (0:w194:dbl)
                            n187 = Equal?(x=w194, y=w193) -> (x = y?=w188:bool)
                            n188 = Equal To 0?(x=w189) -> (x = 0?=w187:bool)
                            n189 = Or(x=w188, y=w187) -> (x .or. y?=w186:bool)
                            n190 = Multiply(x=w184, y=0.25) -> (x*y=w214:dbl)
                            n191 = Select(t=0.985 ("x"), s=w186, f=0.95) -> (s? t:f=w190:dbl)
                            n192 = Add(x=w214, y=w215) -> (x+y=w178:dbl)
                            n193 = Multiply(x=w190, y=w195) -> (x*y=w199:dbl)
                            n194 = Absolute Value(x=w178) -> (abs(x)=w183:dbl)
                            n195 = Add(x=w199, y=w189) -> (x+y=w201:dbl)
                            n196 = Less?(x=w183, y=1e-06) -> (x < y?=w181:bool)
                            n197 = In Range and Coerce(upper limit=w206, x=w201, lower limit=w205) -> (coerced(x)=w200:dbl)  [unwired: 1 out]
                            n198 = feedback-in #3(w200) -> ()
                            n199 = Select(t=0.0, s=w181, f=w178) -> (s? t:f=w179:dbl)
                            n200 = global write "G_VEH.vi" "theta handle"(w179) -> ()
                          }
                          frame Enabled {
                            n201 = flat-sequence {
                              tunnel: [w248] -> w219
                              frame #0 {
                                n202 = global read "G_VEH.vi" "candata"() -> (w247:T8)
                                n203 = Unbundle By Name(w247) -> ("VS_can"=w246:dbl)
                                n204 = Multiply(x=w246, y=0.5) -> (x*y=w244:dbl)
                                n205 = In Range and Coerce(upper limit=50.0, x=w244, lower limit=40.0) -> (coerced(x)=w241:dbl)  [unwired: 1 out]
                                n206 = Multiply(x=w241, y=w241) -> (x*y=w252:dbl)
                                n207 = Multiply(x=w241, y=w252) -> (x*y=w254:dbl)
                                n208 = Multiply(x=w252, y=0.5) -> (x*y=w249:dbl)
                                n209 = Divide(x=w254, y=3.0) -> (x/y=w250:dbl)
                                n210 = Build Array(w250, w249, w241) -> (w248:dbl[])
                              }
                            }
                            n211 = flat-sequence {
                              tunnel: [w231] -> w229
                              frame #0 {
                                n212 = global read "G_SEN.vi" "Lane_L_I"() -> (w236:dbl[])
                                n213 = global read "G_SEN.vi" "Lane_R_I"() -> (w235:dbl[])
                                n214 = Multiply(x=w236, y=0.5) -> (x*y=w239:dbl[])
                                n215 = Multiply(x=w235, y=0.5) -> (x*y=w240:dbl[])
                                n216 = Add(x=w239, y=w240) -> (x+y=w234:dbl[])
                                n217 = global write "G_SEN.vi" "Lane_C_I"(w234) -> ()
                                n218 = Array Subset(array=w234, index=1, length=3) -> (w231:dbl[])
                              }
                            }
                            n219 = Multiply(x=w229, y=w219) -> (x*y=w230:dbl[])
                            n220 = Add Array Elements(numeric array=w230) -> (sum=w228:dbl)
                            n221 = global read "G_VEH.vi" "handle"() -> (w226:dbl)
                            n222 = Multiply(x=-0.2, y=w228) -> (x*y=w225:dbl)
                            n223 = Multiply(x=w225, y=0.1 ("x")) -> (x*y=w223:dbl)
                            n224 = Multiply(x=0.9, y=w226) -> (x*y=w222:dbl)
                            n225 = Add(x=w223, y=w222) -> (x+y=w221:dbl)
                            n226 = global write "G_VEH.vi" "handle"(w221) -> ()
                          }
                        }
                      }
                      frame #2 {
                        n227 = call "collision_fixed_steer.vi"("obsclose"="obs", "Max. Vel."="Max. Vel.") -> ("collision"=w257:bool, "speed limit"=→"Speed limit":dbl)  [unwired: 8 in]
                        "collision" <- w257
                        n228 = Boolean To (0,1)(Boolean=w257) -> (0, 1=→"col":i16)
                      }
                      frame #3 {
                        n229 = global read "G_PATH.vi" "Mission"() -> (w260:i32)
                        "Mission" <- w260
                        n230 = case shown="9" w260 {
                          frame 0, Default {
                          }
                          frame 9 {
                            n231 = flat-sequence {
                              frame #0 {
                                n232 = global write "G_PATH.vi" "parking_cost"(0 ("parkingcost")) -> ()
                                n233 = global write "G_VEH.vi" "xparking"(T9 {"c_idx"=-1, "xc"=0.0, "yc"=0.0, "hc"=0.0, "xc_path"=0.0} ("xparking")) -> ()
                                n234 = global write "G_PATH.vi" "wpt_park"(dbl[][] [] ("wpt_park")) -> ()
                              }
                              frame #1 {
                                n235 = global read "G_PATH.vi" "path_rev"() -> (w264:dbl[][])
                                n236 = Empty Array?(array=w264) -> (empty?=w265:bool)
                                n237 = case shown="False" w265 {
                                frame False {
                                n238 = flat-sequence {
                                frame #0 {
                                n239 = disable-structure shown="Enabled" {
                                frame Enabled {
                                n240 = global read "G_PATH.vi" "path_rev"() -> (w271:dbl[][])
                                n241 = global read "G_VEH.vi" "xyhp"() -> (w266:T5)
                                n242 = Empty Array?(array=w271) -> (empty?=w270:bool)
                                n243 = Unbundle By Name(w266) -> ("idx"=w272:i32)
                                n244 = Not(x=w270) -> (.not. x?=w269:bool)
                                n245 = Equal To 0?(x=w272) -> (x = 0?=w268:bool)
                                n246 = And(x=w269, y=w268) -> (x .and. y?=w267:bool)
                                n247 = case shown="True" w267 {
                                frame False {
                                }
                                frame True {
                                n248 = flat-sequence {
                                tunnel: [w276] -> w273
                                frame #0 {
                                n249 = global read "G_PATH.vi" "path_rev"() -> (w274:dbl[][])
                                n250 = global write "G_PATH.vi" "path"(w274) -> ()
                                n251 = global write "G_PATH.vi" "path_origin"(w274) -> ()
                                }
                                frame #1 {
                                n252 = call "whereami.vi"() -> ()  [unwired: 12 in]
                                }
                                frame #2 {
                                n253 = global read "G_PATH.vi" "path"() -> (w275:dbl[][])
                                n254 = global read "G_VEH.vi" "xyhc"() -> (w277:T5)
                                n255 = call "findcurrentpointinpath.vi"("xyhc_in"=w277, "path_updated"=w275) -> ("xyhc_out"=w276:T5)  [unwired: 8 in, 1 out]
                                }
                                }
                                n256 = global write "G_VEH.vi" "xyhc"(w273) -> ()
                                }
                                }
                                }
                                frame Disabled {
                                }
                                }
                                }
                                frame #1 {
                                n257 = global read "G_VEH.vi" "xparking"() -> (w298:T5)
                                n258 = global read "G_NAV.vi" "M6006"() -> (w297:T7)
                                n259 = Unbundle By Name(w297) -> ("lcc[1]"=w295:dbl, "lcc[0]"=w293:dbl)
                                n260 = Unbundle By Name(w298) -> ("x"=w296:dbl, "y"=w294:dbl)
                                n261 = Subtract(x=w296, y=w295) -> (x-y=w292:dbl)
                                n262 = Subtract(x=w294, y=w293) -> (x-y=w291:dbl)
                                n263 = global read "G_VEH.vi" "candata"() -> (w285:T8)
                                n264 = Square(x=w292) -> (x^2=w290:dbl)
                                n265 = Square(x=w291) -> (x^2=w289:dbl)
                                n266 = Unbundle By Name(w285) -> ("VS_can"=w284:dbl)
                                n267 = Add(x=w290, y=w289) -> (x+y=w288:dbl)
                                n268 = Absolute Value(x=w284) -> (abs(x)=w283:dbl)
                                n269 = Square Root(x=w288) -> (sqrt(x)=w287:dbl)
                                n270 = global read "G_VEH.vi" "firstcall"() -> (w278:bool)
                                n271 = Less?(x=w287, y=1.2) -> (x < y?=w281:bool)
                                n272 = Less?(x=w283, y=0.05) -> (x < y?=w280:bool)
                                n273 = Compound Arithmetic op=AND(w278, w281, w280) -> (w279:bool)
                                n274 = case shown="False" w279 {
                                tunnel: w287 -> [w299 _]
                                frame False {
                                n275 = global read "G_SEN.vi" "sensor_etc"() -> (w302:dbl[][])
                                n276 = global read "G_VEH.vi" "candata"() -> (w309:T8)
                                n277 = Unbundle By Name(w309) -> ("VS_can"=w308:dbl)
                                n278 = Empty Array?(array=w302) -> (empty?=w301:bool)
                                n279 = In Range and Coerce(upper limit=6.0, x=w299, lower limit=1.5) -> (In Range?=w307:bool)  [unwired: 1 out]
                                n280 = Less Or Equal To 0?(x=w308) -> (x <= 0?=w306:bool)
                                n281 = Not(x=w301) -> (.not. x?=w300:bool)
                                n282 = Compound Arithmetic op=AND(w306, w307, w300) -> (w305:bool)
                                n283 = case shown="True" w305 {
                                frame False {
                                }
                                frame True {
                                n284 = global write "G_VEH.vi" "firstcall"(TRUE ("firstcall")) -> ()
                                n285 = call "parking_ung2rev.vi"() -> ()  [unwired: 12 in]
                                }
                                }
                                }
                                frame True {
                                n286 = flat-sequence {
                                frame #0 {
                                n287 = global write "G_VEH.vi" "firstcall"(FALSE ("firstcall")) -> ()
                                n288 = global write "G_VEH.vi" "parking_loop"(TRUE ("parking_loop")) -> ()
                                }
                                frame #1 {
                                n289 = call "parking_ung2_loop.vi"() -> ()  [unwired: 12 in]
                                }
                                }
                                }
                                }
                                }
                                }
                                }
                                frame True {
                                n290 = global read "G_VEH.vi" "xmission"() -> (w326:T5)
                                n291 = global read "G_NAV.vi" "M6006"() -> (w325:T7)
                                n292 = global write "G_VEH.vi" "parking_loop"(FALSE ("parking_loop")) -> ()
                                n293 = global write "G_VEH.vi" "firstcall"(TRUE ("firstcall")) -> ()
                                n294 = Unbundle By Name(w325) -> ("lcc[1]"=w323:dbl, "lcc[0]"=w321:dbl)
                                n295 = Unbundle By Name(w326) -> ("x"=w324:dbl, "y"=w322:dbl)
                                n296 = Subtract(x=w324, y=w323) -> (x-y=w320:dbl)
                                n297 = Subtract(x=w322, y=w321) -> (x-y=w319:dbl)
                                n298 = Square(x=w320) -> (x^2=w318:dbl)
                                n299 = Square(x=w319) -> (x^2=w317:dbl)
                                n300 = Add(x=w318, y=w317) -> (x+y=w316:dbl)
                                n301 = Square Root(x=w316) -> (sqrt(x)=w315:dbl)
                                n302 = Greater?(x=w315, y=5.0) -> (0:w313:bool)
                                n303 = case shown="True" w313 {
                                frame False {
                                }
                                frame True {
                                n304 = call "parking_ung2.vi"() -> ()  [unwired: 12 in]
                                }
                                }
                                }
                                }
                              }
                            }
                          }
                        }
                      }
                    }
                  }
                  frame True {
                    n305 = flat-sequence {
                      frame #0 {
                        w330 = FALSE ("X Scale.Loose Fit")
                        w329 = u8 0 ("X Scale.Scale Fit")
                        n306 = call "initvar.vi"() -> ()  [unwired: 12 in]
                        n307 = property on="XY Graph" class="XYGraph (strict)"("XScale.ScaleFit"=w329, "YScale.ScaleFit"=w329, "XScale.LooseFit"=w330, "YScale.LooseFit"=w330) -> ()  [unwired: 2 in, 2 out]
                      }
                      frame #1 {
                        n308 = global read "G_VEH.vi" "Location"() -> (w331:i32)
                        n309 = Bundle("Minimum"=-22.6, "Minimum"=22.6, "Minimum"=10.0, "Minimum"=1.0, "Minimum"=-20.0) -> (w344:T10)  [unwired: 1 in]
                        n310 = Bundle("Minimum"=-5.0, "Minimum"=37.3, "Minimum"=10.0, "Minimum"=1.0, "Minimum"=-20.0) -> (w337:T10)  [unwired: 1 in]
                        n311 = property on="XY Graph" class="XYGraph (strict)"("XScale.Range"=w344) -> ()  [unwired: 2 in, 2 out]
                        n312 = property on="XY Graph" class="XYGraph (strict)"("YScale.Range"=w337) -> ()  [unwired: 2 in, 2 out]
                        n313 = call "getecefdcmref.vi"("map"=w331) -> ("XYZ"=w332:dbl[])  [unwired: 10 in, 4 out]
                        n314 = global write "G_NAV.vi" "ecef ref"(w332) -> ()
                      }
                      frame #2 {
                        n315 = global read "G_DATA.vi" "path"() -> (w347:path)
                        n316 = Build Path(base path=w347, name or relative path="wpt") -> (appended path=w345:path)
                        n317 = call "Read From Measurement File2"("Filename"=w345, "Reset"=TRUE) -> ("error out"=w349:errorcluster, "Signals"=w351:dynamicdata)  [unwired: 4 in, 4 out]
                        n318 = Unbundle By Name(w349) -> ("status"=w348:bool)
                        n319 = case shown="False" w348 {
                          tunnel: w351 -> [w352 _]
                          frame False {
                            n320 = call "Convert from Dynamic Data2"("Dynamic Data Type"=w352) -> ("Array"=w354:dbl[][])  [unwired: 3 in]
                            n321 = Empty Array?(array=w354) -> (empty?=w353:bool)
                            n322 = case shown="False" w353 {
                              tunnel: w354 -> [w355 _]
                              frame False {
                                n323 = call "path_ini_new.vi"("WPT"=w355) -> ()  [unwired: 11 in]
                              }
                              frame True {
                                w356 = T11 [] ("Missions_origin")
                                w357 = dbl[][] [] ("path_updated")
                                n324 = global write "G_PATH.vi" "path"(w357) -> ()
                                n325 = global write "G_PATH.vi" "path_very_origin"(w357) -> ()
                                n326 = global write "G_PATH.vi" "path_origin"(w357) -> ()
                                n327 = global write "G_PATH.vi" "Missions_origin"(w356) -> ()
                                n328 = global write "G_PATH.vi" "Missions"(w356) -> ()
                              }
                            }
                          }
                          frame True {
                          }
                        }
                      }
                      frame #3 {
                        n329 = disable-structure shown="Enabled" {
                          disable-tunnel: [w359 _] -> w358
                          frame Disabled {
                            n330 = disable-structure shown="Enabled" {
                              disable-tunnel: [w365 _] -> w362
                              disable-tunnel: [w363 errorcluster {"status"=TRUE, "code"=0, "source"=""} ("error out")] -> w361
                              frame Enabled {
                                n331 = call "Read From Measurement File"("Reset"=TRUE) -> ("error out"=w363:errorcluster, "Signals"=w365:dynamicdata)  [unwired: 5 in, 4 out]
                              }
                              frame Disabled {
                              }
                            }
                            n332 = Unbundle By Name(w361) -> ("status"=w360:bool)
                            n333 = case shown="False" w360 {
                              tunnel: w362 -> [w371 _]
                              tunnel: [w367 _] -> w359
                              frame False {
                                n334 = call "Convert from Dynamic Data"("Dynamic Data Type"=w371) -> ("Array"=w368:dbl[][])  [unwired: 3 in]
                                n335 = for {
                                tunnel: w368 -> [w379] mode=indexing
                                tunnel: [w373] -> w369 mode=indexing
                                w372 = T5 {"idx"=0, "x"=0.0, "y"=0.0, "h"=0.0, "x_path"=0.0}  # x
                                n336 = Index Array(array=w379, index #1=0 ("index")) -> (element #1=w377:dbl, element #2=w376:dbl, element #3=w375:dbl)  [unwired: 2 in]
                                n337 = Bundle By Name(cluster=w372, "idx"=w377, "x"=w376, "y"=w375) -> (w374:T5)
                                n338 = Build Cluster Array(w374) -> (w373:T12)
                                }
                                n339 = Index Array(array=w369, index (col)=0 ("disabled index (col)")) -> (element=w367:T12)  [unwired: 1 in]
                              }
                              frame True {
                              }
                            }
                          }
                          frame Enabled {
                          }
                        }
                        n340 = global write "G_PATH.vi" "Missions_origin"(w358) -> ()
                        n341 = global write "G_PATH.vi" "Missions"(w358) -> ()
                      }
                      frame #4 {
                        n342 = local write "Load WPT"(FALSE ("Load WPT")) -> ()
                        n343 = global read "G_VEH.vi" "Location"() -> (w380:i32)
                        n344 = call "mapconf.vi"("Location"=w380) -> ("y"=w382:cluster{dbl, dbl, "y":dbl, "y":dbl, dbl}, "x"=w383:cluster{dbl, dbl, "y":dbl, "y":dbl, dbl}, "new picture"=w384:picture)  [unwired: 8 in]
                        n345 = property on="XY Graph 2" class="XYGraph (strict)"("PlotImages.Back"=w384) -> ()  [unwired: 2 in, 2 out]
                        n346 = property on="XY Graph 2" class="XYGraph (strict)"("XScale.Range"=w383, "YScale.Range"=w382) -> ()  [unwired: 2 in, 2 out]
                      }
                    }
                  }
                }
              }
              frame True {
                n347 = flat-sequence {
                  tunnel: [w391] -> w385
                  tunnel: w385 -> [w480]
                  frame #0 {
                    w386 = 0.0
                    n348 = disable-structure shown="Enabled" {
                      frame Disabled {
                        w387 = TRUE ("X Scale.Loose Fit")
                        w388 = u8 2 ("X Scale.Scale Fit")
                        n349 = property on="XY Graph" class="XYGraph (strict)"("XScale.ScaleFit"=w388, "YScale.ScaleFit"=w388, "XScale.LooseFit"=w387, "YScale.LooseFit"=w387) -> ()  [unwired: 2 in, 2 out]
                      }
                      frame Enabled {
                      }
                    }
                    n350 = global write "G_VEH.vi" "handle"(w386) -> ()
                    n351 = global write "G_VEH.vi" "VS_des"(w386) -> ()
                  }
                  frame #1 {
                    n352 = local read "Make WPT"() -> (w390:bool)
                    n353 = global read "G_VEH.vi" "Location"() -> (w389:i32)
                    n354 = Initialize Array(0.0 ("element"), 7 ("dimension size"), 1 ("dimension size")) -> (w392:dbl[][])
                    n355 = while {
                      shift-right: [w397] -> w391
                      shift-left: w392 -> [w399]
                      shift-right: [FALSE] -> _
                      shift-left: w390 -> [w400]
                      tunnel: w389 -> [w396]
                      stop <- w402 stop-if-true
                      n356 = flat-sequence {
                        tunnel: [w412] -> w398
                        tunnel: w396 -> [w405]
                        frame #0 {
                          n357 = global read "G_NAV.vi" "GPS_status"() -> (w404:T13)
                          n358 = disable-structure shown="Enabled" {
                            disable-tunnel: [w423 w427] -> w415
                            disable-tunnel: [w422 w426] -> w414
                            disable-tunnel: [w416 w425] -> w413
                            disable-tunnel: w404 -> [w421 w435]
                            disable-tunnel: [w420 w434] -> w411
                            disable-tunnel: [w419 w433] -> w410
                            disable-tunnel: [w416 w432] -> w409
                            disable-tunnel: w405 -> [_ w431]
                            frame Enabled {
                              n359 = global read "G_NAV.vi" "M6006"() -> (w424:T7)
                              n360 = Unbundle By Name(w424) -> ("lcc[0]"=w418:dbl, "lcc[1]"=w417:dbl)
                              n361 = Unbundle By Name(w421) -> ("lat"=w420:dbl, "lon"=w419:dbl, "hgt"=w416:dbl)
                              n362 = To Double Precision Float(number=w418) -> (double precision float=w423:dbl)
                              n363 = To Double Precision Float(number=w417) -> (double precision float=w422:dbl)
                            }
                            frame Disabled {
                              n364 = Unbundle By Name(w435) -> ("lat"=w434:dbl, "lon"=w433:dbl, "hgt"=w432:dbl)
                              n365 = call "getecefdcmref.vi"("map"=w431) -> ("XYZ"=w430:dbl[])  [unwired: 10 in, 4 out]
                              n366 = call "llh2lcc.vi"("ecef ref"=w430, "hgt"=w432, "lon"=w433, "lat"=w434) -> ("lcc"=w429:dbl[])  [unwired: 7 in]
                              n367 = Index Array(array=w429, index #1=0 ("index")) -> (element #1=w427:dbl, element #2=w426:dbl, element #3=w425:dbl)  [unwired: 2 in]
                            }
                          }
                          n368 = global read "G_VEH.vi" "candata"() -> (w408:T8)
                          n369 = Unbundle By Name(w408) -> ("VS_can"=w407:dbl)
                          n370 = To Double Precision Float(number=w405) -> (double precision float=w406:dbl)
                          n371 = Build Array(w411, w410, w409, w415, w414, w413, w407, w406) -> (w412:dbl[])
                        }
                      }
                      n372 = local read "Make WPT"() -> (w403:bool)
                      n373 = Not(x=w403) -> (.not. x?=w402:bool)
                      n374 = case shown="False" w400 {
                        tunnel: w399 -> [w450 w467]
                        tunnel: w398 -> [w449 w465]
                        tunnel: [w448 w464] -> w397
                        frame False {
                          n375 = Array Size(array=w450) -> (size(s)=w458:i32[])
                          n376 = Index Array(array=w458, index=1) -> (element=w447:i32)
                          n377 = Decrement(x=w447) -> (x-1=w446:i32)
                          n378 = Index Array(array=w450, index (col)=w446) -> (element=w454:dbl[])  [unwired: 1 in]
                          n379 = Index Array(array=w454, index #1=3 ("index"), index #2=4 ("index")) -> (element #1=w445:dbl, element #2=w443:dbl)
                          n380 = Index Array(array=w449, index #1=3 ("index"), index #2=4 ("index")) -> (element #1=w444:dbl, element #2=w442:dbl)
                          n381 = Subtract(x=w445, y=w444) -> (x-y=w441:dbl)
                          n382 = Subtract(x=w443, y=w442) -> (x-y=w440:dbl)
                          n383 = Square(x=w441) -> (x^2=w439:dbl)
                          n384 = Square(x=w440) -> (x^2=w438:dbl)
                          n385 = Add(x=w439, y=w438) -> (x+y=w437:dbl)
                          n386 = Greater Or Equal?(x=w437, y=0.25) -> (x >= y?=w451:bool)
                          n387 = case shown="True" w451 {
                            tunnel: w450 -> [w459 w463]
                            tunnel: w447 -> [_ w460]
                            tunnel: w449 -> [_ w462]
                            tunnel: [w459 w461] -> w448
                            frame False {
                            }
                            frame True {
                              n388 = Insert Into Array(array=w463, index (col)=w460, new element=w462) -> (w461:dbl[][])  [unwired: 1 in]
                            }
                          }
                        }
                        frame True {
                          n389 = Replace Array Subset(array=w467, new element=w465, index (col)=0 ("disabled index (col)")) -> (w464:dbl[][])  [unwired: 1 in]
                        }
                      }
                    }
                  }
                  frame #2 {
                    n390 = call "Convert to Dynamic Data"("2D Array"=w480) -> ("Dynamic Data Type"=w481:dynamicdata)  [unwired: 3 in]
                    n391 = global read "G_VEH.vi" "Location"() -> (w477:i32)
                    n392 = case shown="9" w477 {
                      tunnel: ["" ("String") "Hyundai" ("String") "KAIST" ("String") "AJOU" ("String") "MUNJI" ("String") "Airforce" ("String") "CAR" ("String") "KATRI" ("String") _ "coex" ("String")] -> w476
                      frame 0, Default {
                      }
                      frame 1 {
                      }
                      frame 2 {
                      }
                      frame 3 {
                      }
                      frame 4 {
                      }
                      frame 5 {
                      }
                      frame 6 {
                      }
                      frame 7 {
                      }
                      frame 8 {
                      }
                      frame 9 {
                      }
                    }
                    n393 = Get Date/Time In Seconds() -> (seconds since 1Jan1904=w478:timestamp)
                    n394 = Format Date/Time String(time format string (%c)="%2y%2m%2d%2H%2M", seconds (now)=w478) -> (date/time string=w474:string)  [unwired: 1 in]
                    n395 = global read "G_DATA.vi" "path"() -> (w472:path)
                    n396 = Build Path(base path=w472, name or relative path="wpt") -> (appended path=w470:path)
                    n397 = Concatenate Strings(w474, "_" ("string"), w476, ".lvm" ("string")) -> (w469:string)
                    n398 = Build Path(base path=w470, name or relative path=w469) -> (appended path=w468:path)
                    n399 = call "save wpt"("Signals"=w481, "Reset"=TRUE, "Filename"=w468) -> ()  [unwired: 14 in, 3 out]
                  }
                }
              }
            }
          }
        }
      }
    }
  }
  n400 = disable-structure shown="Enabled" {
    frame Disabled {
    }
    frame Enabled {
      n401 = while {
        tunnel: [w493] -> w492 mode=indexing
        stop <- "Boolean 2" stop-if-true
        n402 = flat-sequence {
          tunnel: [w498] -> w494
          tunnel: [w508] -> w495
          tunnel: w494 -> [w508]
          tunnel: w495 -> [w541]
          tunnel: [w540] -> w493
          frame #0 {
            n403 = Wait Until Next ms Multiple(millisecond multiple=u32 10) -> ()  [unwired: 1 out]
          }
          frame #1 {
            w499 = TRUE ("Sensor [F12]")
            n404 = call "Ibeopaser.vi"("Hide Transparent"=w499, "Sensor [F12]"=w499) -> ("x_sensor"=w502:T5, "etc"=w500:dbl[][], "lane"=w501:dbl[][], "obs"=w503:dbl[][], "update"=w498:bool)  [unwired: 5 in]
            n405 = case shown="True" w498 {
              tunnel: w503 -> [_ w507]
              tunnel: w502 -> [_ w506]
              tunnel: w501 -> [_ w505]
              tunnel: w500 -> [_ w504]
              frame False {
              }
              frame True {
                n406 = global write "G_SEN.vi" "sensor_obs"(w507) -> ()
                n407 = global write "G_SEN.vi" "sensor_lane"(w505) -> ()
                n408 = global write "G_SEN.vi" "sensor_etc"(w504) -> ()
                n409 = global write "G_VEH.vi" "xsensor"(w506) -> ()
              }
            }
            n410 = call "mobileyepaser.vi"() -> ()  [unwired: 12 in]
            n411 = call "velodynepaser.vi"() -> ()  [unwired: 9 in, 3 out]
          }
          frame #2 {
            n412 = disable-structure shown="Enabled" {
              disable-tunnel: [w510 "Boolean"] -> w509
              frame Disabled {
                n413 = First Call?() -> (First Call?: T/F=w510:bool)
              }
              frame Enabled {
              }
            }
            n414 = case shown="True" w509 {
              frame False {
              }
              frame True {
                n415 = global read "G_SEN.vi" "sensor_obs"() -> (w516:dbl[][])
                n416 = disable-structure shown="Enabled" {
                  disable-tunnel: [w521 T14 [[1.0, 0.0, 0.0, 0.0], [0.0, 1.0, 0.0, 0.0], [0.0, 0.0, 1.0, 0.0], [0.0, 0.0, 0.0, 1.0]] ("pos_slam")] -> w513
                  frame Enabled {
                    w528 = 0.0 ("element")
                    w531 = 0.0 ("element")
                    n417 = global read "G_LCM.vi" "POS_T"() -> (w520:T15)
                    n418 = Unbundle By Name(w520) -> ("heading"=w519:dbl, "y"=w518:dbl, "x"=w517:dbl)
                    n419 = Subtract(x=1.5707963267948966, y=w519) -> (x-y=w537:dbl)
                    n420 = Sine & Cosine(0:w537) -> (1:w534:dbl, 2:w533:dbl)
                    n421 = Negate(x=w534) -> (-x=w536:dbl)
                    n422 = Build Array(w534, w533, 0.0 ("element"), w517) -> (w525:dbl[])
                    n423 = Build Array(w533, w536, 0.0 ("element"), w518) -> (w526:dbl[])
                    n424 = Build Array(w531, w531, 1.0 ("element"), 0.0 ("element")) -> (w524:dbl[])
                    n425 = Build Array(w528, w528, w528, 1.0 ("element")) -> (w523:dbl[])
                    n426 = Build Array(w526, w525, w524, w523) -> (w522:dbl[][])
                    n427 = call-poly <vilib>:"Array To Matrix.vi"("Real 2D Array"=w522) -> ("Real Matrix"=w521:T14)
                  }
                  frame Disabled {
                  }
                }
                n428 = local write "Boolean"(FALSE ("Boolean")) -> ()
                n429 = global write "G_SEN.vi" "sensor_obs_log"(w516) -> ()
                n430 = call-poly <vilib>:"A x B.vi"("B"=w513, "A"=T14 [[1.0, 0.0, 0.0, 0.0], [0.0, 1.0, 0.0, 0.0], [0.0, 0.0, 1.0, 0.0], [0.0, 0.0, 0.0, 1.0]] ("pos_slam")) -> ("A x B"=w512:T14)  [unwired: 1 out]
                n431 = global write "G_VEH.vi" "pos_slam"(w512) -> ()
              }
            }
          }
          frame #3 {
            n432 = disable-structure shown="Enabled" {
              disable-tunnel: w541 -> [w543 _ _]
              disable-tunnel: [w542 _ _] -> w540
              frame Enabled {
                n433 = case shown="True" w543 {
                  tunnel: [_ w545] -> w542
                  frame False {
                  }
                  frame True {
                    n434 = flat-sequence {
                      tunnel: [w563] -> w549
                      tunnel: [w552] -> w548
                      tunnel: [w557] -> w547
                      tunnel: [w555] -> w546
                      tunnel: w549 -> [w609]
                      tunnel: w548 -> [w608]
                      tunnel: w547 -> [w607]
                      tunnel: w546 -> [w603]
                      tunnel: [w602] -> w544
                      tunnel: [w684] -> w545
                      tunnel: w544 -> [w684]
                      frame #0 {
                        w570 = 0.0 ("element")
                        w572 = 0.0 ("element")
                        w573 = 0.0 ("element")
                        n435 = disable-structure shown="Enabled" {
                          disable-tunnel: [w577 w597] -> w561
                          disable-tunnel: [_ w585] -> w559
                          disable-tunnel: [_ w582] -> w560
                          frame Disabled {
                            n436 = global read "G_VEH.vi" "CAN_T_log"() -> (w579:T16)
                            n437 = global read "G_LCM.vi" "CAN_T"() -> (w580:T16)
                            n438 = Subtract(x=w580, y=w579) -> (x-y=w578:T16)
                            n439 = Unbundle By Name(w578) -> ("time"=w577:dbl)
                          }
                          frame Enabled {
                            n440 = global read "G_LCM.vi" "POS_T"() -> (w592:T15)
                            n441 = Unbundle By Name(w592) -> ("sys time"=w601:i64)
                            n442 = feedback-in #5(w592) -> ()
                            n443 = feedback #5(w592) -> (w593:T15)
                            n444 = Unbundle By Name(w593) -> ("sys time"=w600:i64)
                            n445 = Add(x=w593, y=w592) -> (x+y=w596:T15)
                            n446 = Subtract(x=w601, y=w600) -> (x-y=w599:i64)
                            n447 = Multiply(x=w596, y=0.5) -> (x*y=w594:T17)
                            n448 = Unbundle By Name(w594) -> ("speed"=w586:dbl, "yaw_rate"=w591:dbl)
                            n449 = Multiply(x=w599, y=1e-06) -> (x*y=w597:dbl)
                            n450 = Equal To 0?(x=w586) -> (x = 0?=w588:bool)
                            n451 = Negate(x=w591) -> (-x=w589:dbl)
                            n452 = Multiply(x=w586, y=0.984) -> (x*y=w585:dbl)
                            n453 = Add(x=w589, y=-0.00062331) -> (x+y=w587:dbl)
                            n454 = Select(t=w586, s=w588, f=w587) -> (s? t:f=w583:dbl)
                            n455 = Multiply(x=w583, y=1.0) -> (x*y=w582:dbl)
                          }
                        }
                        n456 = Multiply(x=w561, y=w560) -> (x*y=w557:dbl)
                        n457 = Multiply(x=w561, y=w559) -> (x*y=w552:dbl)
                        n458 = Sine & Cosine(0:w557) -> (1:w551:dbl, 2:w554:dbl)
                        n459 = Multiply(x=w554, y=w552) -> (x*y=w553:dbl)
                        n460 = Multiply(x=w552, y=w551) -> (x*y=w550:dbl)
                        n461 = Negate(x=w551) -> (-x=w571:dbl)
                        n462 = Build Array(w554, w551, w572, w572) -> (w569:dbl[])
                        n463 = Build Array(w553, w550, 0.0 ("element"), 1.0 ("element")) -> (w566:dbl[])
                        n464 = Build Array(w571, w554, w570, w570) -> (w568:dbl[])
                        n465 = Build Array(w573, w573, 1.0 ("element"), 0.0 ("element")) -> (w567:dbl[])
                        n466 = Build Array(w569, w568, w567, w566) -> (w565:dbl[][])
                        n467 = Transpose 2D Array(2D array=w565) -> (transposed array=w564:dbl[][])
                        n468 = global read "G_VEH.vi" "pos_slam"() -> (w562:T14)
                        n469 = call-poly <vilib>:"Array To Matrix.vi"("Real 2D Array"=w564) -> ("Real Matrix"=w556:T14)
                        n470 = call-poly <vilib>:"A x B.vi"("B"=w556, "A"=w562) -> ("A x B"=w563:T14)  [unwired: 1 out]
                        n471 = call "mat2pos.vi"("Real Matrix"=w556) -> ("pos"=w555:dbl[])  [unwired: 10 in]
                      }
                      frame #1 {
                        n472 = global read "G_SEN.vi" "sensor_obs_log"() -> (w641:dbl[][])
                        n473 = To Single Precision Float(number=w641) -> (single precision float=w640:sgl[][])
                        n474 = Index Array(array=w640, index (col) #1=1 ("disabled index (col)"), index (col) #2=0 ("index (col)")) -> (element #1=w620:sgl[], element #2=w619:sgl[])  [unwired: 2 in]
                        n475 = Negate(x=w619) -> (-x=w618:sgl[])
                        n476 = disable-structure shown="Enabled" {
                          disable-tunnel: [w659 w667 w669] -> w628
                          disable-tunnel: [w658 w666 w668] -> w627
                          disable-tunnel: w620 -> [w654 w667 w674]
                          disable-tunnel: w618 -> [w653 w666 w673]
                          disable-tunnel: w608 -> [_ _ w671]
                          disable-tunnel: w607 -> [_ _ w670]
                          frame Disabled {
                            n477 = global read "G_VEH.vi" "xsensor_log"() -> (w664:T5)
                            n478 = Unbundle By Name(w664) -> ("x"=w663:dbl, "y"=w662:dbl, "h"=w651:dbl)
                            n479 = global read "G_VEH.vi" "xsensor"() -> (w657:T5)
                            n480 = Subtract(x=1.5707963267948966, y=w651) -> (x-y=w650:dbl)
                            n481 = Unbundle By Name(w657) -> ("x"=w656:dbl, "y"=w655:dbl, "h"=w648:dbl)
                            n482 = call "rotm_mimo.vi"("angle[rad]"=w650, "reverse"=TRUE, "y0"=w662, "x0"=w663, "y"=w653, "x"=w654) -> ("Y"=w661:dbl[], "X"=w660:dbl[])  [unwired: 2 in, 2 out]
                            n483 = Subtract(x=1.5707963267948966, y=w648) -> (x-y=w647:dbl)
                            n484 = call "rotm_mimo.vi"("angle[rad]"=w647, "y0"=w655, "x0"=w656, "y"=w661, "x"=w660) -> ("Y"=w658:dbl[], "X"=w659:dbl[])  [unwired: 3 in, 2 out]
                          }
                          frame Enabled {
                          }
                          frame Disabled {
                            n485 = call "rotm_mimo.vi"("angle[rad]"=w670, "y0"=0.0, "x0"=w671, "y"=w673, "x"=w674) -> ("Y"=w668:dbl[], "X"=w669:dbl[])  [unwired: 3 in, 2 out]
                          }
                        }
                        n486 = global read "G_SEN.vi" "sensor_obs_log"() -> (w625:dbl[][])
                        n487 = global read "G_SEN.vi" "sensor_obs"() -> (w635:dbl[][])
                        n488 = To Single Precision Float(number=w625) -> (single precision float=w626:sgl[][])
                        n489 = To Single Precision Float(number=w635) -> (single precision float=w636:sgl[][])
                        n490 = Index Array(array=w626, index (col)=2 ("disabled index (col)")) -> (element=w623:sgl[])  [unwired: 1 in]
                        n491 = Index Array(array=w636, index (col) #1=1 ("disabled index (col)"), index (col) #2=0 ("index (col)"), index (col) #3=2 ("index (col)")) -> (element #1=w634:sgl[], element #2=w615:sgl[], element #3=w637:sgl[])  [unwired: 3 in]
                        n492 = Negate(x=w615) -> (-x=w614:sgl[])
                        n493 = disable-structure shown="Enabled" {
                          disable-tunnel: [w646 _] -> w638
                          disable-tunnel: w623 -> [w645 _]
                          frame Enabled {
                            n494 = Build Array(w645) -> (w646:sgl[][])
                          }
                          frame Disabled {
                          }
                        }
                        n495 = Build Array(w634) -> (w632:sgl[][])
                        n496 = disable-structure shown="Enabled" {
                          disable-tunnel: w637 -> [w644 _]
                          disable-tunnel: [w643 _] -> w630
                          frame Enabled {
                            n497 = Build Array(w644) -> (w643:sgl[][])
                          }
                          frame Disabled {
                          }
                        }
                        n498 = Build Array(w614) -> (w631:sgl[][])
                        n499 = Build Array(w628) -> (w642:sgl[][])
                        n500 = Build Array(w627) -> (w639:sgl[][])
                        n501 = call "ICP_preALIGNMENT_LV2010.vi"("X_target"=w642, "Y_target"=w639, "icp_maxCorrespondence_distance"=2.0, "Z_target"=w638, "X_source"=w632, "Y_source"=w631, "Z_source"=w630) -> ("transformation_matrix"=w612:sgl[][], "icprot"=w606:sgl[][], "converged?"=w610:bool)  [unwired: 13 in, 5 out]
                        n502 = call-poly <vilib>:"Array To Matrix.vi"("Real 2D Array"=w612) -> ("Real Matrix"=w613:T14)
                        n503 = call-poly <vilib>:"Array To Matrix.vi"("Real 2D Array"=w606) -> ("Real Matrix"=w605:T14)
                        n504 = disable-structure shown="Enabled" {
                          disable-tunnel: [w678 w683] -> w611
                          disable-tunnel: w613 -> [w676 _]
                          disable-tunnel: w609 -> [w677 w683]
                          disable-tunnel: w610 -> [w675 _]
                          frame Disabled {
                            n505 = case shown="True" w675 {
                              tunnel: [w679 w682] -> w678
                              tunnel: w677 -> [w679 w681]
                              tunnel: w676 -> [_ w680]
                              frame False {
                              }
                              frame True {
                                n506 = call-poly <vilib>:"A x B.vi"("B"=w680, "A"=w681) -> ("A x B"=w682:T14)  [unwired: 1 out]
                              }
                            }
                          }
                          frame Enabled {
                          }
                        }
                        n507 = call "mat2pos.vi"("Real Matrix"=w605) -> ("pos"=w604:dbl[])  [unwired: 10 in]
                        n508 = Build Array (concatenate)(w604, w603) -> (w602:dbl[])
                        n509 = global write "G_VEH.vi" "pos_slam"(w611) -> ()
                      }
                      frame #2 {
                        n510 = global read "G_SEN.vi" "sensor_obs"() -> (w685:dbl[][])
                        n511 = global write "G_SEN.vi" "sensor_obs_log"(w685) -> ()
                      }
                    }
                  }
                }
              }
              frame Disabled {
              }
              frame Disabled {
                n512 = global read "G_VEH.vi" "xsensor"() -> (w687:T5)
                n513 = Unbundle By Name(w687) -> ("x"=w688:dbl, "y"=w689:dbl, "h"=w690:dbl)
                n514 = global read "G_SEN.vi" "sensor_obs"() -> (w691:dbl[][])
                n515 = Build Array(w688, w689, w690) -> (w686:dbl[])
                n516 = flat-sequence {
                  tunnel: w691 -> [w693]
                  tunnel: w686 -> [w694]
                  frame #0 {
                    n517 = Empty Array?(array=w693) -> (empty?=w692:bool)
                    n518 = case shown="False" w692 {
                      tunnel: w693 -> [w702 _]
                      tunnel: w694 -> [w696 _]
                      frame False {
                        n519 = flat-sequence {
                          tunnel: w702 -> [w705]
                          tunnel: w696 -> [w704]
                          tunnel: [w703] -> w698
                          tunnel: [w720] -> w697
                          tunnel: w698 -> [w720]
                          tunnel: [w706] -> w695
                          frame #0 {
                            n520 = call "chopdata2.vi"("velo"=w705, "pos"=w704) -> ("slam_pos"=w703:dbl[])  [unwired: 9 in]
                          }
                          frame #1 {
                            w710 = 0 ("disabled index (col)")
                            n521 = global read "G_SEN.vi" "pos_slam"() -> (w719:dbl[][])
                            n522 = Index Array(array=w719, index (row) #1=0 ("index (col)"), index (col) #1=2 ("disabled index (col)"), index (row) #2=1 ("index (row)"), index (col) #2=2 ("disabled index (col)"), index (row) #3=0 ("index (row)"), index (col) #3=1 ("disabled index (col)"), index (row) #4=w710, index (col) #4=w710) -> (element #1=w714:dbl, element #2=w713:dbl, element #3=w709:dbl, element #4=w708:dbl)
                            n523 = Inverse Tangent (2 Input)(1:w708, 2:w709) -> (0:w707:dbl)
                            n524 = Build Array(w714, w713, w707) -> (w706:dbl[])
                          }
                        }
                        n525 = Build Array (concatenate)(w696, w697, w695) -> (w701:dbl[])
                        n526 = local read item#-1() -> (w699)
                        n527 = Build Array (concatenate)(w699, w701) -> (w700:dbl[][])
                      }
                      frame True {
                      }
                    }
                  }
                }
              }
            }
          }
        }
      }
      "Array" <- w492
    }
  }
  n528 = disable-structure shown="Enabled" {
    frame Disabled {
      n529 = flat-sequence {
        frame #0 {
          n530 = local write "obs"(FALSE ("obs")) -> ()
          n531 = local write "log"(TRUE ("obs")) -> ()
        }
        frame #1 {
          n532 = while {
            stop <- FALSE stop-if-true
            n533 = flat-sequence {
              frame #0 {
                n534 = Wait Until Next ms Multiple(millisecond multiple=u32 20 ("milliseconds to wait")) -> (millisecond timer value=w727:u32)
                n535 = feedback #6() -> (w725:u32)  [unwired: 1 in]
                n536 = feedback-in #6(w727) -> ()
                n537 = Subtract(x=w727, y=w725) -> (x-y=→"timmer":u32)
              }
              frame #1 {
                n538 = disable-structure shown="Enabled" {
                  frame Disabled {
                    n539 = Select(t=0.97, s="log", f=0.0) -> (s? t:f=w729:dbl)
                    n540 = call "obslog.vi"("xmax"=8.0, "xmin"=-5.0, "FF"=w729, "ymin"=0.0, "ymax"=20.0) -> ()  [unwired: 7 in]
                  }
                  frame Enabled {
                  }
                }
              }
              frame #2 {
                n541 = disable-structure shown="Enabled" {
                  frame Disabled {
                  }
                  frame Enabled {
                    n542 = disable-structure shown="Enabled" {
                      frame Disabled {
                        n543 = global read "G_PATH.vi" "RXY"() -> (w753:dbl[])
                        n544 = Index Array(array=w753) -> (element=w752:dbl)  [unwired: 1 in]
                        n545 = feedback #7(0.0 ("t")) -> (w744:dbl)
                        n546 = Greater?(x=w752, y=600.0) -> (0:w736:bool)
                        n547 = Multiply(x=0.95, y=w744) -> (x*y=w740:dbl)
                        n548 = Select(s=w736, f=i16 0) -> (s? t:f=w748:i16)  [unwired: 1 in]
                        n549 = Greater?(x=w740, y=0.01) -> (0:w741:bool)
                        n550 = Select(t=w740, s=w741, f=0.0) -> (s? t:f=w738:dbl)
                        n551 = Greater?(x=w748, y=i16 300) -> (0:w747:bool)
                        n552 = Select(t=1.0, s=w747, f=w738) -> (s? t:f=w737:dbl)
                        n553 = feedback-in #7(w737) -> ()
                        n554 = global write "G_SEN.vi" "crosswalk"(w737) -> ()
                      }
                      frame Enabled {
                        n555 = call "lanelog.vi"() -> ()  [unwired: 12 in]
                      }
                    }
                  }
                }
              }
              frame #3 {
                n556 = disable-structure shown="Enabled" {
                  frame Disabled {
                    n557 = global read "G_PATH.vi" "xxx"() -> (w755:dbl)
                    n558 = Equal To 0?(x=w755) -> (x = 0?=w754:bool)
                    n559 = case shown="True" w754 {
                      frame False {
                      }
                      frame True {
                        n560 = call "lane.vi"("predict"=TRUE) -> ()  [unwired: 11 in]
                      }
                    }
                  }
                  frame Enabled {
                  }
                }
              }
            }
          }
        }
      }
    }
    frame Enabled {
      n561 = flat-sequence {
        frame #0 {
          n562 = for {
            N: 500 -> [_]
            tunnel: [w761] -> w760 mode=indexing
            i -> [w764]
            n563 = To Double Precision Float(number=w764) -> (double precision float=w763:dbl)
            n564 = Multiply(x=0.1, y=w763) -> (x*y=w761:dbl)
          }
          n565 = global write "G_SEN.vi" "keydata"(dbl[][] [] ("keydata")) -> ()
          n566 = global write "G_VEH.vi" "pos_slam"(T14 [[1.0, 0.0, 0.0, 0.0], [0.0, 1.0, 0.0, 0.0], [0.0, 0.0, 1.0, 0.0], [0.0, 0.0, 0.0, 1.0]] ("pos_slam")) -> ()
          n567 = global write "G_SEN.vi" "y_mobileye"(w760) -> ()
        }
        frame #1 {
          n568 = while {
            stop <- FALSE stop-if-true
            n569 = flat-sequence {
              frame #0 {
                n570 = Wait Until Next ms Multiple(millisecond multiple=u32 10) -> ()  [unwired: 1 out]
              }
              frame #1 {
                n571 = global read "G_VEH.vi" "xsensor"() -> (w778:T5)
                n572 = feedback-in #8(w778) -> ()
                n573 = feedback #8(T5 {"idx"=0, "x"=0.0, "y"=0.0, "h"=0.0, "x_path"=0.0} ("xsensor")) -> (w779:T5)
                n574 = global read "G_VEH.vi" "candata"() -> (w775:T8)
                n575 = global read "G_LCM.vi" "POS_T"() -> (w769:T15)
                n576 = Not Equal?(x=w778, y=w779) -> (x != y?=w777:T18)
                n577 = Unbundle By Name(w775) -> ("VS_can"=w774:dbl)
                n578 = Unbundle By Name(w769) -> ("dt"=w768:dbl)
                n579 = Cluster To Array(cluster=w777) -> (array=w776:bool[])
                n580 = Or Array Elements(Boolean array=w776) -> (logical OR=w772:bool)
                n581 = Greater Than 0?(x=w768) -> (x > 0?=w767:bool)
                n582 = Greater?(x=w774, y=1.0) -> (0:w771:bool)
                n583 = Compound Arithmetic op=AND(w772, w771, w767) -> (w770:bool)
                n584 = case shown="True" w770 {
                  frame False {
                  }
                  frame True {
                    n585 = flat-sequence {
                      frame #0 {
                      }
                      frame #1 {
                        n586 = flat-sequence {
                          frame #0 {
                            n587 = global read "G_SEN.vi" "sensor_lane_log"() -> (w815:dbl[][])
                            n588 = global read "G_SEN.vi" "sensor_lane"() -> (w816:dbl[][])
                            n589 = global read "G_VEH.vi" "xsensor"() -> (w813:T5)
                            n590 = call "sensor_log.vi"("xsensor"=w813, "sensor_log"=w815, "sensor"=w816) -> ("sensor_log_out"=w814:dbl[][])  [unwired: 6 in, 2 out]
                            n591 = global write "G_SEN.vi" "sensor_lane_log"(w814) -> ()
                          }
                        }
                        n592 = global read "G_SEN.vi" "sensor_lane"() -> (w791:dbl[][])
                        n593 = global read "G_SEN.vi" "sensor_lane"() -> (w792:dbl[][])
                        n594 = global read "G_SEN.vi" "lane_log_R"() -> (w806:dbl[][])
                        n595 = global read "G_SEN.vi" "lane_log_L"() -> (w803:dbl[][])
                        n596 = global read "G_SEN.vi" "Lane_L_M"() -> (w785:dbl[])
                        n597 = global read "G_SEN.vi" "Lane_R_M"() -> (w786:dbl[])
                        n598 = global read "G_VEH.vi" "xsensor"() -> (w788:T5)
                        n599 = global read "G_VEH.vi" "xsensor"() -> (w787:T5)
                        n600 = call "lanelog2.vi"("xsensor"=w788, "thresh"=0.02, "lane_log"=w803, "sensor"=w791, "Lane_M"=w785) -> ("lane_log_out"=w804:dbl[][], "sensor_out"=w782:dbl[][], "lane_I_out"=w789:dbl[])  [unwired: 2 in, 2 out]
                        n601 = call "lanelog2.vi"("xsensor"=w787, "thresh"=0.02, "lane_log"=w806, "sensor"=w792, "Lane_M"=w786) -> ("lane_log_out"=w805:dbl[][], "sensor_out"=w781:dbl[][], "lane_I_out"=w790:dbl[])  [unwired: 2 in, 2 out]
                        n602 = disable-structure shown="Disabled" {
                          disable-tunnel: w782 -> [w808 _]
                          frame Disabled {
                            n603 = call "Convert to Dynamic Data2"("2D Array"=w808) -> ("Dynamic Data Type"=w809:dynamicdata)  [unwired: 3 in]
                            n604 = call "Write To Measurement File"("Signals"=w809, "Filename"=path "left.lvm") -> ()  [unwired: 15 in, 3 out]
                          }
                          frame Enabled {
                          }
                        }
                        n605 = global write "G_SEN.vi" "lane_log_L"(w804) -> ()
                        n606 = disable-structure shown="Disabled" {
                          disable-tunnel: w781 -> [w810 _]
                          frame Disabled {
                            n607 = call "Convert to Dynamic Data3"("2D Array"=w810) -> ("Dynamic Data Type"=w811:dynamicdata)  [unwired: 3 in]
                            n608 = call "Write To Measurement File2"("Signals"=w811, "Filename"=path "right.lvm") -> ()  [unwired: 15 in, 3 out]
                          }
                          frame Enabled {
                          }
                        }
                        n609 = global write "G_SEN.vi" "lane_log_R"(w805) -> ()
                        n610 = Index Array(array=w789, index=0) -> (element=w800:dbl)
                        n611 = Index Array(array=w790, index=0) -> (element=w801:dbl)
                        n612 = Not Equal To 0?(x=w800) -> (x != 0?=w797:bool)
                        n613 = Not Equal To 0?(x=w801) -> (x != 0?=w798:bool)
                        n614 = Build Array(w798, w797) -> (w796:bool[])
                        n615 = Boolean Array To Number(Boolean array=w796) -> (number=w795:u32)
                        n616 = case shown="3" w795 {
                          tunnel: w790 -> [_ w857 _ w958]
                          tunnel: w789 -> [_ _ w899 w959]
                          tunnel: [w818 w856 w897 w950] -> w784
                          tunnel: [w817 w855 w898 w940] -> w783
                          frame 0, Default {
                            n617 = flat-sequence {
                              tunnel: [w819] -> w817
                              frame #0 {
                                w832 = 0.0 ("element")
                                n618 = global read "G_SEN.vi" "lane_width"() -> (w831:dbl)
                                n619 = global read "G_SEN.vi" "Lane_L_I"() -> (w825:dbl[])
                                n620 = Multiply(x=w831, y=-0.5) -> (x*y=w829:dbl)
                                n621 = Array Subset(array=w825, index=0, length=4) -> (w824:dbl[])
                                n622 = Build Array(w832, w832, w832, w829) -> (w828:dbl[])
                                n623 = global read "G_SEN.vi" "Lane_L_I"() -> (w823:dbl[])
                                n624 = Multiply(x=w824, y=0.975) -> (x*y=w834:dbl[])
                                n625 = Multiply(x=w828, y=0.025) -> (x*y=w833:dbl[])
                                n626 = Add(x=w834, y=w833) -> (x+y=w821:dbl[])
                                n627 = Array Subset(array=w823, index=4) -> (w820:dbl[])  [unwired: 1 in]
                                n628 = Build Array (concatenate)(w821, w820) -> (w819:dbl[])
                              }
                            }
                            n629 = flat-sequence {
                              tunnel: [w837] -> w818
                              frame #0 {
                                w850 = 0.0 ("element")
                                n630 = global read "G_SEN.vi" "lane_width"() -> (w851:dbl)
                                n631 = global read "G_SEN.vi" "Lane_R_I"() -> (w843:dbl[])
                                n632 = Multiply(x=w851, y=0.5) -> (x*y=w853:dbl)
                                n633 = Array Subset(array=w843, index=0, length=4) -> (w842:dbl[])
                                n634 = Build Array(w850, w850, w850, w853) -> (w854:dbl[])
                                n635 = global read "G_SEN.vi" "Lane_R_I"() -> (w841:dbl[])
                                n636 = Multiply(x=w842, y=0.975) -> (x*y=w848:dbl[])
                                n637 = Multiply(x=w854, y=0.025) -> (x*y=w849:dbl[])
                                n638 = Add(x=w848, y=w849) -> (x+y=w839:dbl[])
                                n639 = Array Subset(array=w841, index=4) -> (w838:dbl[])  [unwired: 1 in]
                                n640 = Build Array (concatenate)(w839, w838) -> (w837:dbl[])
                              }
                            }
                          }
                          frame 1 {
                            n641 = flat-sequence {
                              tunnel: w857 -> [w892]
                              tunnel: [w880] -> w856
                              frame #0 {
                                n642 = global read "G_SEN.vi" "Lane_R_I"() -> (w889:dbl[])
                                n643 = global read "G_VEH.vi" "xsensor"() -> (w887:T5)
                                n644 = To Double Precision Float(number=w887) -> (double precision float=w886:T19)
                                n645 = Array Subset(array=w889, index=0, length=4) -> (w888:dbl[])
                                n646 = Cluster To Array(cluster=w886) -> (array=w885:dbl[])
                                n647 = Multiply(x=w888, y=0.6) -> (x*y=w894:dbl[])
                                n648 = Multiply(x=w892, y=0.4) -> (x*y=w893:dbl[])
                                n649 = Add(x=w894, y=w893) -> (x+y=w881:dbl[])
                                n650 = Array Subset(array=w885, index=1, length=3) -> (w882:dbl[])
                                n651 = Build Array (concatenate)(w881, w882) -> (w880:dbl[])
                              }
                            }
                            n652 = flat-sequence {
                              tunnel: w857 -> [w872]
                              tunnel: [w858] -> w855
                              frame #0 {
                                n653 = global read "G_SEN.vi" "lane_width"() -> (w877:dbl)
                                n654 = Index Array(array=w872, index=3) -> (element=w878:dbl)
                                n655 = Subtract(x=w878, y=w877) -> (x-y=w875:dbl)
                                n656 = global read "G_SEN.vi" "Lane_L_I"() -> (w862:dbl[])
                                n657 = Replace Array Subset(array=w872, new element #1=w875, index #1=3 ("index"), new element #2=0.25 ("new element/subarray"), index #2=0 ("index")) -> (w867:dbl[])
                                n658 = Array Subset(array=w862, index=0, length=4) -> (w864:dbl[])
                                n659 = global read "G_SEN.vi" "Lane_L_I"() -> (w859:dbl[])
                                n660 = Multiply(x=w864, y=0.6) -> (x*y=w870:dbl[])
                                n661 = Multiply(x=w867, y=0.4) -> (x*y=w871:dbl[])
                                n662 = Add(x=w870, y=w871) -> (x+y=w861:dbl[])
                                n663 = Array Subset(array=w859, index=4) -> (w860:dbl[])  [unwired: 1 in]
                                n664 = Build Array (concatenate)(w861, w860) -> (w858:dbl[])
                              }
                            }
                          }
                          frame 2 {
                            n665 = flat-sequence {
                              tunnel: w899 -> [w914]
                              tunnel: [w900] -> w897
                              frame #0 {
                                n666 = global read "G_SEN.vi" "lane_width"() -> (w919:dbl)
                                n667 = Index Array(array=w914, index=3) -> (element=w920:dbl)
                                n668 = Add(x=w920, y=w919) -> (x+y=w917:dbl)
                                n669 = global read "G_SEN.vi" "Lane_R_I"() -> (w907:dbl[])
                                n670 = Replace Array Subset(array=w914, new element #1=w917, index #1=3 ("index"), new element #2=0.25 ("new element/subarray"), index #2=0 ("index")) -> (w909:dbl[])
                                n671 = Array Subset(array=w907, index=0, length=4) -> (w905:dbl[])
                                n672 = global read "G_SEN.vi" "Lane_R_I"() -> (w904:dbl[])
                                n673 = Multiply(x=w905, y=0.6) -> (x*y=w911:dbl[])
                                n674 = Multiply(x=w909, y=0.4) -> (x*y=w910:dbl[])
                                n675 = Add(x=w911, y=w910) -> (x+y=w901:dbl[])
                                n676 = Array Subset(array=w904, index=4) -> (w902:dbl[])  [unwired: 1 in]
                                n677 = Build Array (concatenate)(w901, w902) -> (w900:dbl[])
                              }
                            }
                            n678 = flat-sequence {
                              tunnel: w899 -> [w934]
                              tunnel: [w922] -> w898
                              frame #0 {
                                n679 = global read "G_SEN.vi" "Lane_L_I"() -> (w931:dbl[])
                                n680 = global read "G_VEH.vi" "xsensor"() -> (w929:T5)
                                n681 = To Double Precision Float(number=w929) -> (double precision float=w928:T19)
                                n682 = Array Subset(array=w931, index=0, length=4) -> (w930:dbl[])
                                n683 = Cluster To Array(cluster=w928) -> (array=w927:dbl[])
                                n684 = Multiply(x=w930, y=0.6) -> (x*y=w936:dbl[])
                                n685 = Multiply(x=w934, y=0.4) -> (x*y=w935:dbl[])
                                n686 = Add(x=w936, y=w935) -> (x+y=w924:dbl[])
                                n687 = Array Subset(array=w927, index=1, length=3) -> (w923:dbl[])
                                n688 = Build Array (concatenate)(w924, w923) -> (w922:dbl[])
                              }
                            }
                          }
                          frame 3 {
                            n689 = Subtract(x=w958, y=w959) -> (x-y=w961:dbl[])
                            n690 = Index Array(array=w961, index=3) -> (element=w956:dbl)
                            n691 = Greater?(x=w956, y=2.0) -> (0:w955:bool)
                            n692 = case shown="False" w955 {
                              tunnel: w959 -> [w971 w997]
                              tunnel: [w970 w989] -> w941
                              tunnel: w958 -> [w964 w991]
                              tunnel: [w963 w987] -> w951
                              tunnel: w956 -> [w962 _]
                              frame True {
                                n693 = global write "G_SEN.vi" "lane_width"(w962) -> ()
                                n694 = global read "G_SEN.vi" "Lane_R_I"() -> (w965:dbl[])
                                n695 = global read "G_SEN.vi" "Lane_L_I"() -> (w972:dbl[])
                                n696 = Multiply(x=w972, y=0.6) -> (x*y=w974:dbl[])
                                n697 = Multiply(x=w971, y=0.4) -> (x*y=w973:dbl[])
                                n698 = Multiply(x=w965, y=0.6) -> (x*y=w967:dbl[])
                                n699 = Multiply(x=w964, y=0.4) -> (x*y=w966:dbl[])
                                n700 = Add(x=w974, y=w973) -> (x+y=w970:dbl[])
                                n701 = Add(x=w967, y=w966) -> (x+y=w963:dbl[])
                              }
                              frame False {
                                n702 = global read "G_SEN.vi" "Lane_R_I"() -> (w992:dbl[])
                                n703 = global read "G_SEN.vi" "Lane_L_I"() -> (w998:dbl[])
                                n704 = Multiply(x=w998, y=0.6) -> (x*y=w1000:dbl[])
                                n705 = Multiply(x=w997, y=0.4) -> (x*y=w999:dbl[])
                                n706 = Multiply(x=w992, y=0.6) -> (x*y=w994:dbl[])
                                n707 = Multiply(x=w991, y=0.4) -> (x*y=w993:dbl[])
                                n708 = Add(x=w1000, y=w999) -> (x+y=w977:dbl[])
                                n709 = Add(x=w994, y=w993) -> (x+y=w986:dbl[])
                                n710 = Index Array(array=w977, index=0) -> (element=w980:dbl)
                                n711 = Index Array(array=w986, index=0) -> (element=w984:dbl)
                                n712 = Max & Min(x=w980, y=0.5 ("new element/subarray")) -> (min(x,y)=w978:dbl)  [unwired: 1 out]
                                n713 = Max & Min(x=w984, y=0.5 ("new element/subarray")) -> (min(x,y)=w982:dbl)  [unwired: 1 out]
                                n714 = Replace Array Subset(array=w977, new element=w978, index=0) -> (w989:dbl[])
                                n715 = Replace Array Subset(array=w986, new element=w982, index=0) -> (w987:dbl[])
                              }
                            }
                            n716 = global read "G_VEH.vi" "xsensor"() -> (w949:T5)
                            n717 = To Double Precision Float(number=w949) -> (double precision float=w948:T19)
                            n718 = Cluster To Array(cluster=w948) -> (array=w947:dbl[])
                            n719 = Array Subset(array=w951, index=0, length=4) -> (w952:dbl[])
                            n720 = Array Subset(array=w941, index=0, length=4) -> (w944:dbl[])
                            n721 = Array Subset(array=w947, index=1, length=3) -> (w939:dbl[])
                            n722 = Build Array (concatenate)(w952, w939) -> (w950:dbl[])
                            n723 = Build Array (concatenate)(w944, w939) -> (w940:dbl[])
                          }
                        }
                        n724 = global write "G_SEN.vi" "Lane_R_I"(w784) -> ()
                        n725 = global write "G_SEN.vi" "Lane_L_I"(w783) -> ()
                      }
                      frame #2 {
                        n726 = stacked-sequence {
                          frame #0 {
                            n727 = global read "G_SEN.vi" "Lane_R_I"() -> (w1005:dbl[])
                            n728 = Array Subset(array=w1005, index=0, length=4) -> (w1004:dbl[])
                            n729 = while {
                              shift-right: [w1077] -> _
                              shift-left: dbl[] [] ("lane_I_out") -> [w1076]
                              shift-right: [w1067] -> w1018
                              shift-left: 0 ("size") -> [w1074]
                              shift-right: [w1072] -> w1017
                              shift-left: w1004 -> [w1073]
                              stop <- w1068 stop-if-true
                              n730 = Index Array(array=w1073, index=3) -> (element=w1085:dbl)
                              n731 = Add(x=w1085, y=0.5) -> (x+y=w1081:dbl)
                              n732 = global read "G_SEN.vi" "sensor_obs"() -> (w1089:dbl[][])
                              n733 = global read "G_VEH.vi" "xsensor"() -> (w1066:T5)
                              n734 = Replace Array Subset(array=w1073, new element=w1081, index=3) -> (w1087:dbl[])
                              n735 = call "lanelog2.vi"("xsensor"=w1066, "thresh"=0.025, "lane_log"=dbl[][] [], "sensor"=w1089, "Lane_M"=w1087) -> ("lane_I_out"=w1078:dbl[], "lane_M_out"=w1072:dbl[], "size"=w1075:i32)  [unwired: 2 in, 2 out]
                              n736 = Greater?(x=w1075, y=w1074) -> (0:w1079:bool)
                              n737 = Max & Min(x=w1075, y=w1074) -> (max(x,y)=w1067:i32)  [unwired: 1 out]
                              n738 = Select(t=w1078, s=w1079, f=w1076) -> (s? t:f=w1077:dbl[])
                              n739 = Greater?(x=w1081, y=8.0) -> (0:w1069:bool)
                              n740 = Greater?(x=w1067, y=50) -> (0:w1070:bool)
                              n741 = Or(x=w1069, y=w1070) -> (x .or. y?=w1068:bool)
                            }
                            n742 = flat-sequence {
                              tunnel: [w1055] -> w1016
                              tunnel: [w1054] -> w1015
                              tunnel: w1004 -> [w1052]
                              tunnel: [w1051] -> w1003
                              frame #0 {
                                n743 = global read "G_SEN.vi" "lane_width"() -> (w1060:dbl)
                                n744 = Index Array(array=w1052, index=3) -> (element=w1061:dbl)
                                n745 = Add(x=w1061, y=w1060) -> (x+y=w1058:dbl)
                                n746 = global read "G_SEN.vi" "lane_log_RR"() -> (w1056:dbl[][])
                                n747 = global read "G_SEN.vi" "sensor_lane"() -> (w1065:dbl[][])
                                n748 = global read "G_VEH.vi" "xsensor"() -> (w1053:T5)
                                n749 = Replace Array Subset(array=w1052, new element=w1058, index=3) -> (w1063:dbl[])
                                n750 = call "lanelog2.vi"("xsensor"=w1053, "thresh"=0.025, "lane_log"=w1056, "sensor"=w1065, "Lane_M"=w1063) -> ("lane_log_out"=w1057:dbl[][], "sensor_out"=w1051:dbl[][], "lane_I_out"=w1055:dbl[], "size"=w1054:i32)  [unwired: 2 in, 1 out]
                                n751 = global write "G_SEN.vi" "lane_log_RR"(w1057) -> ()
                              }
                            }
                            n752 = disable-structure shown="Enabled" {
                              disable-tunnel: w1018 -> [w1034 w1050]
                              disable-tunnel: [w1032 w1036] -> w1009
                              disable-tunnel: w1017 -> [w1026 w1043]
                              disable-tunnel: w1016 -> [w1025 w1038]
                              disable-tunnel: w1015 -> [_ w1041]
                              frame Disabled {
                                n753 = Index Array(array=w1026, index=3) -> (element=w1029:dbl)
                                n754 = Index Array(array=w1025, index=3) -> (element=w1028:dbl)
                                n755 = Less?(x=w1029, y=w1028) -> (x < y?=w1027:bool)
                                n756 = Select(t=w1026, s=w1027, f=w1025) -> (s? t:f=w1024:dbl[])
                                n757 = Greater?(x=w1034, y=50) -> (0:w1033:bool)
                                n758 = Select(t=w1024, s=w1033, f=w1025) -> (s? t:f=w1032:dbl[])
                              }
                              frame Enabled {
                                n759 = Greater?(x=w1041, y=w1050) -> (0:w1049:bool)
                                n760 = Index Array(array=w1038, index=3) -> (element=w1046:dbl)
                                n761 = Index Array(array=w1043, index=3) -> (element=w1045:dbl)
                                n762 = Less?(x=w1046, y=w1045) -> (x < y?=w1044:bool)
                                n763 = Select(t=w1038, s=w1044, f=w1043) -> (s? t:f=w1042:dbl[])
                                n764 = Select(t=w1038, s=w1049, f=w1042) -> (s? t:f=w1037:dbl[])
                                n765 = Greater?(x=w1041, y=50) -> (0:w1039:bool)
                                n766 = Select(t=w1038, s=w1039, f=w1037) -> (s? t:f=w1036:dbl[])
                              }
                            }
                            n767 = disable-structure shown="Disabled" {
                              disable-tunnel: w1003 -> [w1021 _]
                              frame Disabled {
                                n768 = call "Convert to Dynamic Data4"("2D Array"=w1021) -> ("Dynamic Data Type"=w1023:dynamicdata)  [unwired: 3 in]
                                n769 = call "Write To Measurement File3"("Signals"=w1023, "Filename"=path "right2.lvm") -> ()  [unwired: 15 in, 3 out]
                              }
                              frame Enabled {
                              }
                            }
                            n770 = global read "G_SEN.vi" "Lane_RR_I"() -> (w1010:dbl[])
                            n771 = Multiply(x=w1010, y=0.8) -> (x*y=w1012:dbl[])
                            n772 = Multiply(x=w1009, y=0.2) -> (x*y=w1011:dbl[])
                            n773 = Add(x=w1012, y=w1011) -> (x+y=w1008:dbl[])
                            n774 = global write "G_SEN.vi" "Lane_RR_I"(w1008) -> ()
                          }
                          frame #1 {
                            n775 = global read "G_SEN.vi" "Lane_L_I"() -> (w1092:dbl[])
                            n776 = Array Subset(array=w1092, index=0, length=4) -> (w1091:dbl[])
                            n777 = while {
                              shift-right: [w1164] -> _
                              shift-left: dbl[] [] ("lane_I_out") -> [w1163]
                              shift-right: [w1154] -> w1105
                              shift-left: 0 ("size") -> [w1161]
                              shift-right: [w1159] -> w1104
                              shift-left: w1091 -> [w1160]
                              stop <- w1155 stop-if-true
                              n778 = Index Array(array=w1160, index=3) -> (element=w1172:dbl)
                              n779 = Subtract(x=w1172, y=0.5) -> (x-y=w1168:dbl)
                              n780 = global read "G_SEN.vi" "sensor_obs"() -> (w1176:dbl[][])
                              n781 = global read "G_VEH.vi" "xsensor"() -> (w1153:T5)
                              n782 = Replace Array Subset(array=w1160, new element=w1168, index=3) -> (w1174:dbl[])
                              n783 = call "lanelog2.vi"("xsensor"=w1153, "thresh"=0.025, "lane_log"=dbl[][] [], "sensor"=w1176, "Lane_M"=w1174) -> ("lane_I_out"=w1165:dbl[], "lane_M_out"=w1159:dbl[], "size"=w1162:i32)  [unwired: 2 in, 2 out]
                              n784 = Greater?(x=w1162, y=w1161) -> (0:w1166:bool)
                              n785 = Max & Min(x=w1162, y=w1161) -> (max(x,y)=w1154:i32)  [unwired: 1 out]
                              n786 = Select(t=w1165, s=w1166, f=w1163) -> (s? t:f=w1164:dbl[])
                              n787 = Less?(x=w1168, y=-8.0) -> (x < y?=w1156:bool)
                              n788 = Greater?(x=w1154, y=50) -> (0:w1157:bool)
                              n789 = Or(x=w1156, y=w1157) -> (x .or. y?=w1155:bool)
                            }
                            n790 = flat-sequence {
                              tunnel: [w1142] -> w1103
                              tunnel: [w1141] -> w1102
                              tunnel: w1091 -> [w1139]
                              tunnel: [w1138] -> w1090
                              frame #0 {
                                n791 = global read "G_SEN.vi" "lane_width"() -> (w1147:dbl)
                                n792 = Index Array(array=w1139, index=3) -> (element=w1148:dbl)
                                n793 = Subtract(x=w1148, y=w1147) -> (x-y=w1145:dbl)
                                n794 = global read "G_SEN.vi" "lane_log_LL"() -> (w1143:dbl[][])
                                n795 = global read "G_SEN.vi" "sensor_lane"() -> (w1152:dbl[][])
                                n796 = global read "G_VEH.vi" "xsensor"() -> (w1140:T5)
                                n797 = Replace Array Subset(array=w1139, new element=w1145, index=3) -> (w1150:dbl[])
                                n798 = call "lanelog2.vi"("xsensor"=w1140, "thresh"=0.025, "lane_log"=w1143, "sensor"=w1152, "Lane_M"=w1150) -> ("lane_log_out"=w1144:dbl[][], "sensor_out"=w1138:dbl[][], "lane_I_out"=w1142:dbl[], "size"=w1141:i32)  [unwired: 2 in, 1 out]
                                n799 = global write "G_SEN.vi" "lane_log_LL"(w1144) -> ()
                              }
                            }
                            n800 = disable-structure shown="Enabled" {
                              disable-tunnel: w1105 -> [w1121 w1137]
                              disable-tunnel: [w1119 w1123] -> w1098
                              disable-tunnel: w1104 -> [w1113 w1130]
                              disable-tunnel: w1103 -> [w1112 w1125]
                              disable-tunnel: w1102 -> [_ w1128]
                              frame Disabled {
                                n801 = Index Array(array=w1113, index=3) -> (element=w1116:dbl)
                                n802 = Index Array(array=w1112, index=3) -> (element=w1115:dbl)
                                n803 = Greater?(x=w1116, y=w1115) -> (0:w1114:bool)
                                n804 = Select(t=w1113, s=w1114, f=w1112) -> (s? t:f=w1111:dbl[])
                                n805 = Greater?(x=w1121, y=50) -> (0:w1120:bool)
                                n806 = Select(t=w1111, s=w1120, f=w1112) -> (s? t:f=w1119:dbl[])
                              }
                              frame Enabled {
                                n807 = Greater?(x=w1128, y=w1137) -> (0:w1136:bool)
                                n808 = Index Array(array=w1125, index=3) -> (element=w1133:dbl)
                                n809 = Index Array(array=w1130, index=3) -> (element=w1132:dbl)
                                n810 = Greater?(x=w1133, y=w1132) -> (0:w1131:bool)
                                n811 = Select(t=w1125, s=w1131, f=w1130) -> (s? t:f=w1129:dbl[])
                                n812 = Select(t=w1125, s=w1136, f=w1129) -> (s? t:f=w1124:dbl[])
                                n813 = Greater?(x=w1128, y=50) -> (0:w1126:bool)
                                n814 = Select(t=w1125, s=w1126, f=w1124) -> (s? t:f=w1123:dbl[])
                              }
                            }
                            n815 = disable-structure shown="Disabled" {
                              disable-tunnel: w1090 -> [w1108 _]
                              frame Disabled {
                                n816 = call "Convert to Dynamic Data5"("2D Array"=w1108) -> ("Dynamic Data Type"=w1109:dynamicdata)  [unwired: 3 in]
                                n817 = call "Write To Measurement File4"("Signals"=w1109, "Filename"=path "left2.lvm") -> ()  [unwired: 15 in, 3 out]
                              }
                              frame Enabled {
                              }
                            }
                            n818 = global read "G_SEN.vi" "Lane_LL_I"() -> (w1101:dbl[])
                            n819 = Multiply(x=w1101, y=0.8) -> (x*y=w1097:dbl[])
                            n820 = Multiply(x=w1098, y=0.2) -> (x*y=w1096:dbl[])
                            n821 = Add(x=w1097, y=w1096) -> (x+y=w1095:dbl[])
                            n822 = global write "G_SEN.vi" "Lane_LL_I"(w1095) -> ()
                          }
                        }
                      }
                    }
                  }
                }
              }
            }
          }
        }
      }
    }
  }
